vi "ABB Load-Save results.vi"(9 "confirm save":bool, 10 "Path":path, 11 "Mode":enum16{"LOAD", "Save"}(ring)) -> ()   [LabVIEW 2017]
uses:
  ABB global.vi
panel:
  in  "Case Constant\n(See Context Help)":bool=TRUE
  out "Categories":string[](array[string])
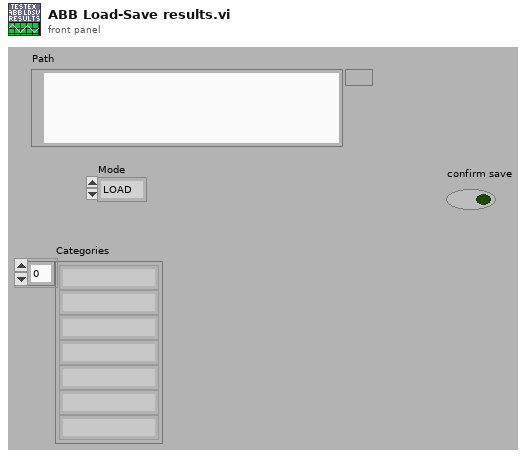
[diagram p1: front panel]
types:
  T1 = cluster{"Stator R":dbl, "Stator dT":dbl, "Rotor R":dbl, "Rotor dT":dbl, "Stator Cooling curve":dbl[][], "Rotor Cooling curve":dbl[][], "Select Resistance":enum16{"Fitted zero Res.", "Selected Res.", "Entered Res."}}
  T2 = cluster{"Stator R":dbl, "Stator dT":dbl, "Rotor R":dbl, "Rotor dT":dbl, "Stator Cooling curve":dbl[][], "Rotor Cooling curve":dbl[][], "Select Resistance":enum16{"Fitted zero Res.", "Selected Res.", "Entered Res."}}[]
  T3 = cluster{"[0]":dbl, "[1]":dbl, "[2]":dbl, "[3]":dbl, "[4]":dbl, "[5]":dbl, "[6]":dbl, "[7]":dbl}
  T4 = cluster{"DBL Array out[0]":dbl, "DBL Array out[1]":dbl, "DBL Array out[2]":dbl}
  T5 = cluster{"VT Primary":dbl, "VT Secondary":dbl, "CT  Primary":dbl, "CT Secondary":dbl, "Current Shunt":enum16{"Internal", "External"}, "Averaging interval":dbl}
  T6 = cluster{"VT Primary":dbl, "VT Secondary":dbl, "CT  Primary":dbl, "CT Secondary":dbl, "Current Shunt":enum16{"Internal", "External"}, "Avg interval":dbl}
  T7 = cluster{"temp. alloc":i32[], "category":i32[], "Category names":string[], "Category none names":string[]}
  T8 = cluster{"Number of Loads":i32, "Loads (%Rated)":dbl[]}
  T9 = enum16{"Fitted zero Res.", "Selected Res.", "Entered Res."}
  T10 = cluster{"Prior to test":dbl, "Prior v":dbl, "Prior temp":dbl, "After test":dbl, "after v":dbl, "After temp":dbl, "Test Voltage (kV)":dbl, "Test Time (min)":dbl}
  T11 = cluster{"Noise Before":string, "Noise During":string}
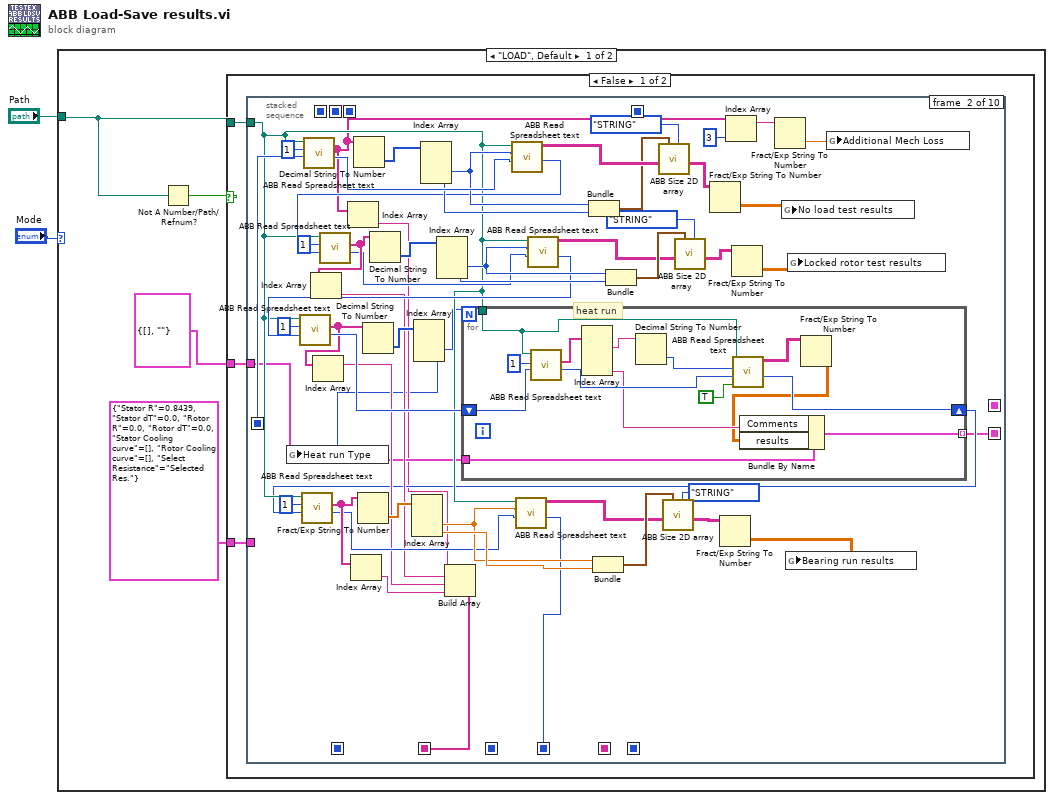
[diagram p0: block diagram]
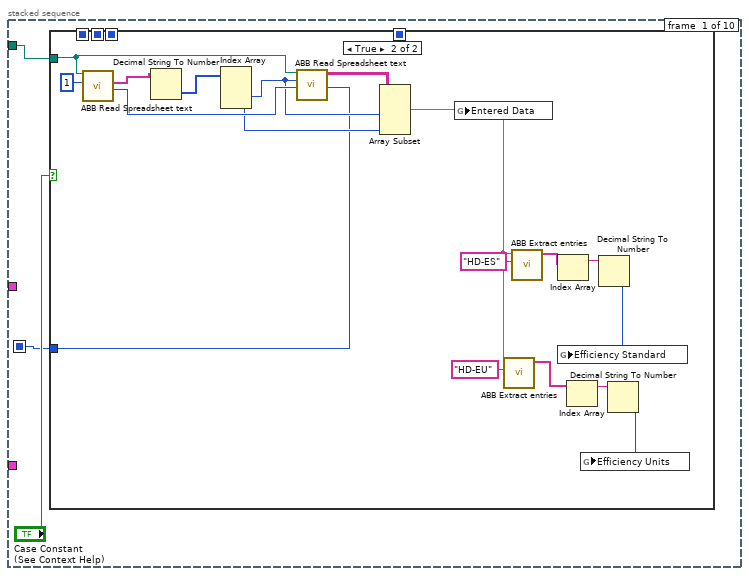
[diagram p2: hidden frame]
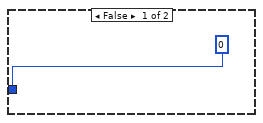
[diagram p3: hidden frame]
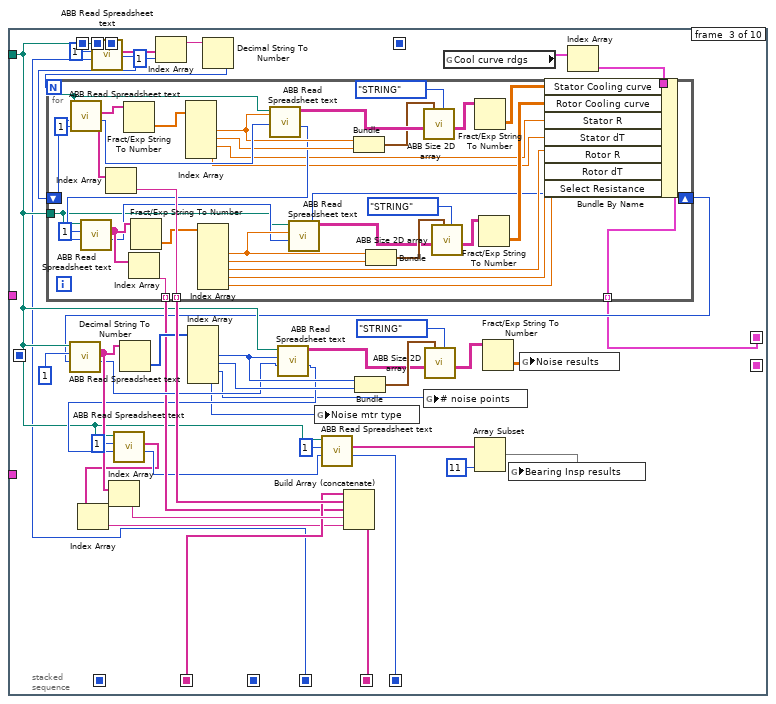
[diagram p4: hidden frame]
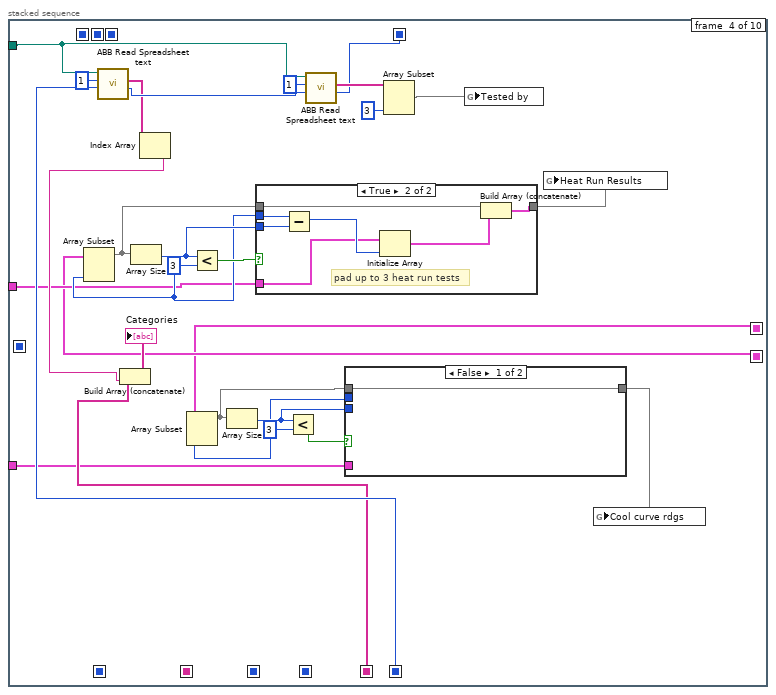
[diagram p5: hidden frame]
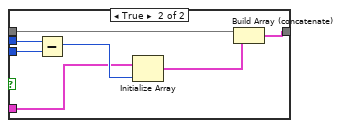
[diagram p6: hidden frame]
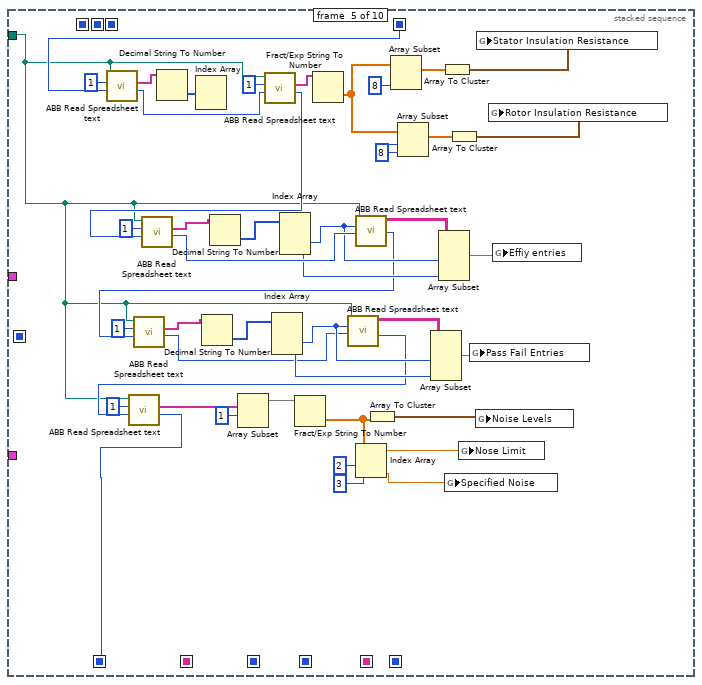
[diagram p8: hidden frame]
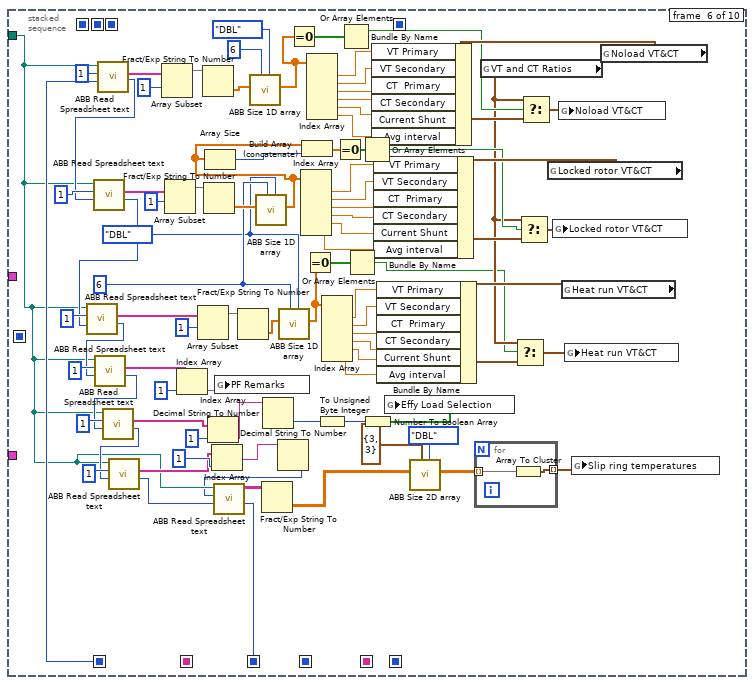
[diagram p9: hidden frame]
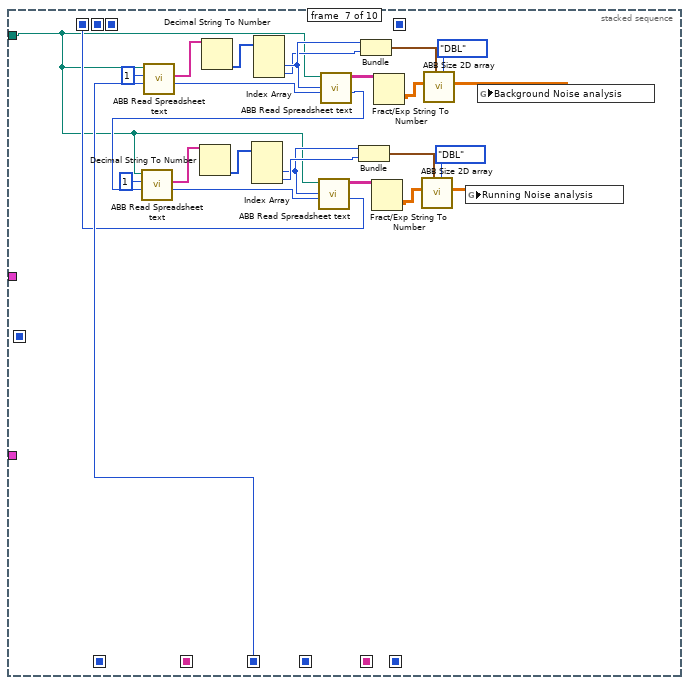
[diagram p10: hidden frame]
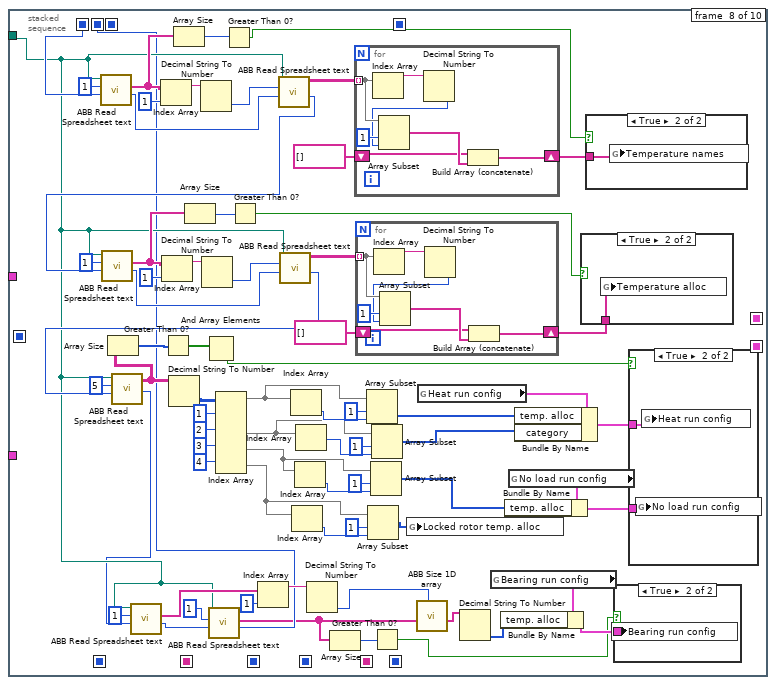
[diagram p11: hidden frame]
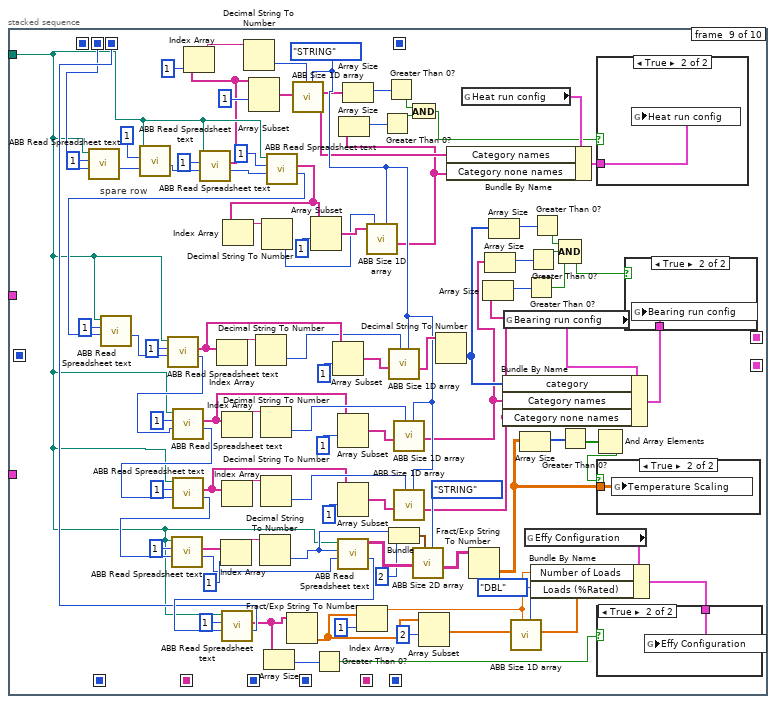
[diagram p16: hidden frame]
diagram:
  n1 = case shown="\"LOAD\", Default" "Mode" {
    tunnel: "Path" -> [w5 w638]
    frame "LOAD", Default {
      n2 = Not A Number/Path/Refnum?(number/path/refnum=w5) -> (NaN/Path/Refnum?=w6:bool)
      n3 = case shown="False" w6 {
        tunnel: w5 -> [w9 _]
        tunnel: cluster{"results":dbl[][], "Comments":string} {"results"=[], "Comments"=""} ("Heat Run") -> [w8 _]
        tunnel: T1 {"Stator R"=0.8439, "Stator dT"=0.0, "Rotor R"=0.0, "Rotor dT"=0.0, "Stator Cooling curve"=[], "Rotor Cooling curve"=[], "Select Resistance"=enum."Selected Res."} ("Cool Curve Rdgs") -> [w7 _]
        frame False {
          n4 = stacked-sequence {
            seq-local: [_ w45 _ _ _ _ _ _ _ _] -> [_ _ w111 _ _ _ _ _ _ _]
            seq-local: [_ w42 _ _ _ _ _ _ _ _] -> [_ _ w126 _ _ _ _ _ _ _]
            seq-local: [w10 _ _ _ _ _ _ _ _ _] -> [_ w75 _ _ _ _ _ _ _ _]
            seq-local: [_ _ w116 _ _ _ _ _ _ _] -> [_ _ _ w200 _ _ _ _ _ _]
            seq-local: [_ _ w114 _ _ _ _ _ _ _] -> [_ _ _ w198 _ _ _ _ _ _]
            seq-local: [_ w38 _ _ _ _ _ _ _ _] -> [_ _ _ w183 _ _ _ _ _ _]
            seq-local: [_ _ _ w182 _ _ _ _ _ _] -> [_ _ _ _ w259 _ _ _ _ _]
            seq-local: [_ _ w102 _ _ _ _ _ _ _] -> [_ _ _ w179 _ _ _ _ _ _]
            seq-local: [_ _ _ _ w223 _ _ _ _ _] -> [_ _ _ _ _ w341 _ _ _ _]
            seq-local: [_ _ _ _ _ w263 _ _ _ _] -> [_ _ _ _ _ _ w378 _ _ _]
            seq-local: [_ _ _ _ _ _ w355 _ _ _] -> [_ _ _ _ _ _ _ w407 _ _]
            seq-local: [_ _ _ _ _ _ _ w384 _ _] -> [_ _ _ _ _ _ _ _ w477 _]
            seq-local: [_ _ _ _ _ _ _ _ w503 _] -> [_ _ _ _ _ _ _ _ _ w591]
            tunnel: w9 -> [w12 w41 w112 w199 w224 w272 w354 w386 w476 w580]
            tunnel: w8 -> [_ w39 _ w184 _ _ _ _ _ _]
            tunnel: w7 -> [_ _ _ w181 _ _ _ _ _ _]
            frame #0 {
              n5 = case shown="True" "Case Constant\n(See Context Help)" {
                tunnel: [0 ("mark after read (chars.)") w23] -> w10
                tunnel: w12 -> [_ w29]
                frame False {
                }
                frame True {
                  n6 = call "ABB Read Spreadsheet text.vi"("number of rows (all:-1)"=1, "file path (dialog if empty)"=w29) -> ("mark after read (chars.)"=w30:i32, "first row"=w28:string[])  [unwired: 5 in, 3 out]
                  n7 = Decimal String To Number(string=w28) -> (number=w27:i32[])  [unwired: 2 in, 1 out]
                  n8 = Index Array(array=w27) -> (element #2=w24:i32, element #3=w25:i32)  [unwired: 3 in, 1 out]
                  n9 = call "ABB Read Spreadsheet text.vi"("start of read offset (chars.:0 )"=w30, "number of rows (all:-1)"=w24, "file path (dialog if empty)"=w29) -> ("mark after read (chars.)"=w23:i32, "all rows"=w26:string[][])  [unwired: 4 in, 3 out]
                  n10 = Array Subset(array=w26, length (row)=w24, length (col)=w25) -> (w17:string[][])  [unwired: 2 in]
                  n11 = global write "ABB global.vi" "Entered Data"(w17) -> ()
                  n12 = call "ABB Extract entries.vi"("Entry ID"="HD-EU", "Entry table in"=w17) -> ("Selected Entries"=w15:string[])  [unwired: 9 in]
                  n13 = call "ABB Extract entries.vi"("Entry ID"="HD-ES", "Entry table in"=w17) -> ("Selected Entries"=w21:string[])  [unwired: 9 in]
                  n14 = Index Array(array=w21) -> (element=w20:string)  [unwired: 1 in]
                  n15 = Index Array(array=w15) -> (element=w16:string)  [unwired: 1 in]
                  n16 = Decimal String To Number(string=w20) -> (number=w19:i32)  [unwired: 2 in, 1 out]
                  n17 = global write "ABB global.vi" "Efficiency Standard"(w19) -> ()
                  n18 = Decimal String To Number(string=w16) -> (number=w14:i32)  [unwired: 2 in, 1 out]
                  n19 = global write "ABB global.vi" "Efficiency Units"(w14) -> ()
                }
              }
            }
            frame #1 {
              n20 = call "ABB Read Spreadsheet text.vi"("start of read offset (chars.:0 )"=w75, "number of rows (all:-1)"=1, "file path (dialog if empty)"=w41) -> ("mark after read (chars.)"=w82:i32, "first row"=w35:string[])  [unwired: 4 in, 3 out]
              n21 = Index Array(array=w35) -> (element=w37:string)  [unwired: 1 in]
              n22 = Decimal String To Number(string=w35) -> (number=w81:i32[])  [unwired: 2 in, 1 out]
              n23 = Index Array(array=w81) -> (element #2=w80:i32, element #3=w79:i32)  [unwired: 3 in, 1 out]
              n24 = call "ABB Read Spreadsheet text.vi"("start of read offset (chars.:0 )"=w82, "number of rows (all:-1)"=w80, "file path (dialog if empty)"=w41) -> ("mark after read (chars.)"=w47:i32, "all rows"=w84:string[][])  [unwired: 4 in, 3 out]
              n25 = call "ABB Read Spreadsheet text.vi"("start of read offset (chars.:0 )"=w47, "number of rows (all:-1)"=1, "file path (dialog if empty)"=w41) -> ("mark after read (chars.)"=w67:i32, "first row"=w72:string[])  [unwired: 4 in, 3 out]
              n26 = Index Array(array=w72) -> (element=w43:string)  [unwired: 1 in]
              n27 = Decimal String To Number(string=w72) -> (number=w68:i32[])  [unwired: 2 in, 1 out]
              n28 = Index Array(array=w68) -> (element #2=w69:i32, element #3=w70:i32)  [unwired: 3 in, 1 out]
              n29 = call "ABB Read Spreadsheet text.vi"("start of read offset (chars.:0 )"=w67, "number of rows (all:-1)"=w69, "file path (dialog if empty)"=w41) -> ("mark after read (chars.)"=w46:i32, "all rows"=w65:string[][])  [unwired: 4 in, 3 out]
              n30 = call "ABB Read Spreadsheet text.vi"("start of read offset (chars.:0 )"=w46, "number of rows (all:-1)"=1, "file path (dialog if empty)"=w41) -> ("mark after read (chars.)"=w62:i32, "first row"=w60:string[])  [unwired: 4 in, 3 out]
              n31 = Index Array(array=w60) -> (element=w44:string)  [unwired: 1 in]
              n32 = Decimal String To Number(string=w60) -> (number=w61:i32[])  [unwired: 2 in, 1 out]
              n33 = Index Array(array=w61) -> (element #2=w36:i32)  [unwired: 3 in, 2 out]
              n34 = global write "ABB global.vi" "Heat run Type"(w36) -> ()
              n35 = for {
                N: w36 -> [_]
                tunnel: w41 -> [w98]
                shift-right: [w90] -> w40
                shift-left: w62 -> [w99]
                tunnel: w39 -> [w97]
                tunnel: [w89] -> w38 mode=indexing
                # "heat run"
                n36 = call "ABB Read Spreadsheet text.vi"("start of read offset (chars.:0 )"=w99, "number of rows (all:-1)"=1, "file path (dialog if empty)"=w98) -> ("mark after read (chars.)"=w95:i32, "first row"=w91:string[])  [unwired: 4 in, 3 out]
                n37 = Index Array(array=w91) -> (element #1=w94:string, element #4=w92:string)  [unwired: 4 in, 2 out]
                n38 = Decimal String To Number(string=w94) -> (number=w93:i32)  [unwired: 2 in, 1 out]
                n39 = call "ABB Read Spreadsheet text.vi"("remove trailng empty strings"=TRUE, "start of read offset (chars.:0 )"=w95, "number of rows (all:-1)"=w93, "file path (dialog if empty)"=w98) -> ("mark after read (chars.)"=w90:i32, "all rows"=w88:string[][])  [unwired: 3 in, 3 out]
                n40 = Fract/Exp String To Number(string=w88) -> (number=w86:dbl[][])  [unwired: 3 in, 1 out]
                n41 = Bundle By Name(cluster=w97, "Comments"=w92, "results"=w86) -> (w89:cluster{"results":dbl[][], "Comments":string})
              }
              n42 = call "ABB Read Spreadsheet text.vi"("start of read offset (chars.:0 )"=w40, "number of rows (all:-1)"=1, "file path (dialog if empty)"=w41) -> ("mark after read (chars.)"=w51:i32, "first row"=w56:string[])  [unwired: 4 in, 3 out]
              n43 = Index Array(array=w56) -> (element=w57:string)  [unwired: 1 in]
              n44 = Fract/Exp String To Number(string=w56) -> (number=w52:dbl[])  [unwired: 3 in, 1 out]
              n45 = Index Array(array=w52) -> (element #2=w53:dbl, element #3=w54:dbl)  [unwired: 3 in, 1 out]
              n46 = Build Array(w37, w43, w44, w57) -> (w42:string[])
              n47 = call "ABB Read Spreadsheet text.vi"("start of read offset (chars.:0 )"=w51, "number of rows (all:-1)"=w53, "file path (dialog if empty)"=w41) -> ("mark after read (chars.)"=w45:i32, "all rows"=w49:string[][])  [unwired: 4 in, 3 out]
              n48 = Bundle(w80, w79) -> (w83:cluster{i32, i32})  [unwired: 1 in]
              n49 = Bundle(w53, w54) -> (w50:cluster{dbl, dbl})  [unwired: 1 in]
              n50 = Bundle(w69, w70) -> (w66:cluster{i32, i32})  [unwired: 1 in]
              n51 = call "ABB Size 2D array.vi"("Type"=enum16{"Integer", "DBL", "STRING", "BOOLEAN"}."STRING", "Size"=w83, "String Array in"=w84) -> ("String Array out"=w76:string[][])  [unwired: 5 in, 3 out]
              n52 = call "ABB Size 2D array.vi"("Type"=enum16{"Integer", "DBL", "STRING", "BOOLEAN"}."STRING", "Size"=w50, "String Array in"=w49) -> ("String Array out"=w59:string[][])  [unwired: 5 in, 3 out]
              n53 = call "ABB Size 2D array.vi"("Type"=enum16{"Integer", "DBL", "STRING", "BOOLEAN"}."STRING", "Size"=w66, "String Array in"=w65) -> ("String Array out"=w74:string[][])  [unwired: 5 in, 3 out]
              n54 = Fract/Exp String To Number(string=w76) -> (number=w77:dbl[][])  [unwired: 3 in, 1 out]
              n55 = Fract/Exp String To Number(string=w59) -> (number=w58:dbl[][])  [unwired: 3 in, 1 out]
              n56 = Index Array(array=w35, index=3) -> (element=w33:string)
              n57 = Fract/Exp String To Number(string=w74) -> (number=w73:dbl[][])  [unwired: 3 in, 1 out]
              n58 = Fract/Exp String To Number(string=w33) -> (number=w32:dbl)  [unwired: 3 in, 1 out]
              n59 = global write "ABB global.vi" "No load test results"(w77) -> ()
              n60 = global write "ABB global.vi" "Bearing run results"(w58) -> ()
              n61 = global write "ABB global.vi" "Locked rotor test results"(w73) -> ()
              n62 = global write "ABB global.vi" "Additional Mech Loss"(w32) -> ()
            }
            frame #2 {
              n63 = call "ABB Read Spreadsheet text.vi"("start of read offset (chars.:0 )"=w111, "number of rows (all:-1)"=1, "file path (dialog if empty)"=w112) -> ("mark after read (chars.)"=w110:i32, "first row"=w108:string[])  [unwired: 4 in, 3 out]
              n64 = Index Array(array=w108, index=1) -> (element=w106:string)
              n65 = Decimal String To Number(string=w106) -> (number=w105:i32)  [unwired: 2 in, 1 out]
              n66 = global read "ABB global.vi" "Cool curve rdgs"() -> (w104:T2)
              n67 = Index Array(array=w104) -> (element=w103:T1)  [unwired: 1 in]
              n68 = for {
                N: w105 -> [_]
                tunnel: [w166] -> w139 mode=indexing
                tunnel: [w152] -> w125 mode=indexing
                tunnel: w103 -> [w145]
                tunnel: [w144] -> w102 mode=indexing
                tunnel: w112 -> [w143]
                shift-right: [w141] -> w109
                shift-left: w110 -> [w142]
                n69 = call "ABB Read Spreadsheet text.vi"("start of read offset (chars.:0 )"=w142, "number of rows (all:-1)"=1, "file path (dialog if empty)"=w143) -> ("mark after read (chars.)"=w171:i32, "first row"=w164:string[])  [unwired: 4 in, 3 out]
                n70 = Index Array(array=w164) -> (element=w166:string)  [unwired: 1 in]
                n71 = Fract/Exp String To Number(string=w164) -> (number=w170:dbl[])  [unwired: 3 in, 1 out]
                n72 = Index Array(array=w170) -> (element #2=w169:dbl, element #3=w168:dbl, element #4=w149:dbl, element #5=w148:dbl)  [unwired: 5 in, 1 out]
                n73 = call "ABB Read Spreadsheet text.vi"("start of read offset (chars.:0 )"=w171, "number of rows (all:-1)"=w169, "file path (dialog if empty)"=w143) -> ("mark after read (chars.)"=w153:i32, "all rows"=w173:string[][])  [unwired: 4 in, 3 out]
                n74 = call "ABB Read Spreadsheet text.vi"("start of read offset (chars.:0 )"=w153, "number of rows (all:-1)"=1, "file path (dialog if empty)"=w143) -> ("mark after read (chars.)"=w157:i32, "first row"=w163:string[])  [unwired: 4 in, 3 out]
                n75 = Index Array(array=w163) -> (element=w152:string)  [unwired: 1 in]
                n76 = Fract/Exp String To Number(string=w163) -> (number=w158:dbl[])  [unwired: 3 in, 1 out]
                n77 = Index Array(array=w158) -> (element #2=w159:dbl, element #3=w160:dbl, element #4=w147:dbl, element #5=w146:dbl, element #6=w140:dbl)  [unwired: 6 in, 1 out]
                n78 = call "ABB Read Spreadsheet text.vi"("start of read offset (chars.:0 )"=w157, "number of rows (all:-1)"=w159, "file path (dialog if empty)"=w143) -> ("mark after read (chars.)"=w141:i32, "all rows"=w155:string[][])  [unwired: 4 in, 3 out]
                n79 = Bundle(w169, w168) -> (w172:cluster{dbl, dbl})  [unwired: 1 in]
                n80 = Bundle(w159, w160) -> (w156:cluster{dbl, dbl})  [unwired: 1 in]
                n81 = call "ABB Size 2D array.vi"("Type"=enum16{"Integer", "DBL", "STRING", "BOOLEAN"}."STRING", "Size"=w172, "String Array in"=w173) -> ("String Array out"=w165:string[][])  [unwired: 5 in, 3 out]
                n82 = call "ABB Size 2D array.vi"("Type"=enum16{"Integer", "DBL", "STRING", "BOOLEAN"}."STRING", "Size"=w156, "String Array in"=w155) -> ("String Array out"=w162:string[][])  [unwired: 5 in, 3 out]
                n83 = Fract/Exp String To Number(string=w165) -> (number=w151:dbl[][])  [unwired: 3 in, 1 out]
                n84 = Fract/Exp String To Number(string=w162) -> (number=w150:dbl[][])  [unwired: 3 in, 1 out]
                n85 = Bundle By Name(cluster=w145, "Stator Cooling curve"=w151, "Rotor Cooling curve"=w150, "Stator R"=w149, "Stator dT"=w148, "Rotor R"=w147, "Rotor dT"=w146, "Select Resistance"=w140) -> (w144:T1)
              }
              n86 = call "ABB Read Spreadsheet text.vi"("start of read offset (chars.:0 )"=w109, "number of rows (all:-1)"=1, "file path (dialog if empty)"=w112) -> ("mark after read (chars.)"=w131:i32, "first row"=w138:string[])  [unwired: 4 in, 3 out]
              n87 = Index Array(array=w138) -> (element=w127:string)  [unwired: 1 in]
              n88 = Decimal String To Number(string=w138) -> (number=w132:i32[])  [unwired: 2 in, 1 out]
              n89 = Index Array(array=w132) -> (element #2=w133:i32, element #3=w134:i32, element #4=w100:i32, element #5=w101:i32)  [unwired: 5 in, 1 out]
              n90 = call "ABB Read Spreadsheet text.vi"("start of read offset (chars.:0 )"=w131, "number of rows (all:-1)"=w133, "file path (dialog if empty)"=w112) -> ("mark after read (chars.)"=w123:i32, "all rows"=w129:string[][])  [unwired: 4 in, 3 out]
              n91 = call "ABB Read Spreadsheet text.vi"("start of read offset (chars.:0 )"=w123, "number of rows (all:-1)"=1, "file path (dialog if empty)"=w112) -> ("mark after read (chars.)"=w122:i32, "first row"=w118:string[])  [unwired: 4 in, 3 out]
              n92 = Index Array(array=w118) -> (element=w117:string)  [unwired: 1 in]
              n93 = global write "ABB global.vi" "Noise mtr type"(w101) -> ()
              n94 = call "ABB Read Spreadsheet text.vi"("start of read offset (chars.:0 )"=w122, "number of rows (all:-1)"=1, "file path (dialog if empty)"=w112) -> ("mark after read (chars.)"=w116:i32, "first row"=w120:string[])  [unwired: 4 in, 3 out]
              n95 = Build Array (concatenate)(w126, w139, w125, w127, w117) -> (w114:string[])
              n96 = Bundle(w133, w134) -> (w130:cluster{i32, i32})  [unwired: 1 in]
              n97 = global write "ABB global.vi" "# noise points"(w100) -> ()
              n98 = call "ABB Size 2D array.vi"("Type"=enum16{"Integer", "DBL", "STRING", "BOOLEAN"}."STRING", "Size"=w130, "String Array in"=w129) -> ("String Array out"=w137:string[][])  [unwired: 5 in, 3 out]
              n99 = Array Subset(array=w120, length=11) -> (w121:string[])  [unwired: 1 in]
              n100 = Fract/Exp String To Number(string=w137) -> (number=w136:dbl[][])  [unwired: 3 in, 1 out]
              n101 = global write "ABB global.vi" "Bearing Insp results"(w121) -> ()
              n102 = global write "ABB global.vi" "Noise results"(w136) -> ()
            }
            frame #3 {
              w175 = 3 ("y")
              w185 = 3 ("y")
              n103 = Array Subset(array=w183, length=w185) -> (w188:cluster{"results":dbl[][], "Comments":string}[])  [unwired: 1 in]
              n104 = call "ABB Read Spreadsheet text.vi"("start of read offset (chars.:0 )"=w200, "number of rows (all:-1)"=1, "file path (dialog if empty)"=w199) -> ("mark after read (chars.)"=w201:i32, "first row"=w197:string[])  [unwired: 4 in, 3 out]
              n105 = Array Size(array=w188) -> (size(s)=w186:i32)
              n106 = Index Array(array=w197) -> (element=w196:string)  [unwired: 1 in]
              n107 = Build Array (concatenate)(w198, w196) -> (→"Categories":string[])
              n108 = Array Subset(array=w179, length=w175) -> (w178:T2)  [unwired: 1 in]
              n109 = Less?(x=w186, y=w185) -> (x < y?=w189:bool)
              n110 = Array Size(array=w178) -> (size(s)=w176:i32)
              n111 = case shown="True" w189 {
                tunnel: w188 -> [w210 w217]
                tunnel: [w210 w212] -> w187
                tunnel: w186 -> [_ w215]
                tunnel: w185 -> [_ w216]
                tunnel: w184 -> [_ w211]
                frame False {
                }
                frame True {
                  # "pad up to 3 heat run tests"
                  n112 = Subtract(x=w216, y=w215) -> (x-y=w214:i32)
                  n113 = Initialize Array(w211, w214) -> (w213:cluster{"results":dbl[][], "Comments":string}[])
                  n114 = Build Array (concatenate)(w217, w213) -> (w212:cluster{"results":dbl[][], "Comments":string}[])
                }
              }
              n115 = Less?(x=w176, y=w175) -> (x < y?=w177:bool)
              n116 = call "ABB Read Spreadsheet text.vi"("start of read offset (chars.:0 )"=w201, "number of rows (all:-1)"=1, "file path (dialog if empty)"=w199) -> ("mark after read (chars.)"=w182:i32, "first row"=w192:string[])  [unwired: 4 in, 3 out]
              n117 = case shown="False" w177 {
                tunnel: w178 -> [w202 w209]
                tunnel: [w202 w204] -> w180
                tunnel: w176 -> [_ w207]
                tunnel: w175 -> [_ w208]
                tunnel: w181 -> [_ w203]
                frame False {
                }
                frame True {
                  n118 = Subtract(x=w208, y=w207) -> (x-y=w206:i32)
                  n119 = Initialize Array(w203, w206) -> (w205:T2)
                  n120 = Build Array (concatenate)(w209, w205) -> (w204:T2)
                }
              }
              n121 = Array Subset(array=w192, length=3) -> (w190:string[])  [unwired: 1 in]
              n122 = global write "ABB global.vi" "Tested by"(w190) -> ()
              n123 = global write "ABB global.vi" "Heat Run Results"(w187) -> ()
              n124 = global write "ABB global.vi" "Cool curve rdgs"(w180) -> ()
            }
            frame #4 {
              w226 = 8 ("length")
              n125 = call "ABB Read Spreadsheet text.vi"("start of read offset (chars.:0 )"=w259, "number of rows (all:-1)"=1, "file path (dialog if empty)"=w224) -> ("mark after read (chars.)"=w258:i32, "first row"=w262:string[])  [unwired: 4 in, 3 out]
              n126 = Decimal String To Number(string=w262) -> (number=w261:i32[])  [unwired: 2 in, 1 out]
              n127 = Index Array(array=w261) -> ()  [unwired: 2 in, 2 out]
              n128 = call "ABB Read Spreadsheet text.vi"("start of read offset (chars.:0 )"=w258, "number of rows (all:-1)"=1, "file path (dialog if empty)"=w224) -> ("mark after read (chars.)"=w247:i32, "first row"=w256:string[])  [unwired: 4 in, 3 out]
              n129 = call "ABB Read Spreadsheet text.vi"("start of read offset (chars.:0 )"=w247, "number of rows (all:-1)"=1, "file path (dialog if empty)"=w224) -> ("mark after read (chars.)"=w254:i32, "first row"=w253:string[])  [unwired: 4 in, 3 out]
              n130 = Decimal String To Number(string=w253) -> (number=w252:i32[])  [unwired: 2 in, 1 out]
              n131 = Index Array(array=w252) -> (element #2=w249:i32, element #3=w250:i32)  [unwired: 3 in, 1 out]
              n132 = Fract/Exp String To Number(string=w256) -> (number=w227:dbl[])  [unwired: 3 in, 1 out]
              n133 = call "ABB Read Spreadsheet text.vi"("start of read offset (chars.:0 )"=w254, "number of rows (all:-1)"=w249, "file path (dialog if empty)"=w224) -> ("mark after read (chars.)"=w238:i32, "all rows"=w251:string[][])  [unwired: 4 in, 3 out]
              n134 = call "ABB Read Spreadsheet text.vi"("start of read offset (chars.:0 )"=w238, "number of rows (all:-1)"=1, "file path (dialog if empty)"=w224) -> ("mark after read (chars.)"=w240:i32, "first row"=w241:string[])  [unwired: 4 in, 3 out]
              n135 = Decimal String To Number(string=w241) -> (number=w242:i32[])  [unwired: 2 in, 1 out]
              n136 = Index Array(array=w242) -> (element #2=w245:i32, element #3=w244:i32)  [unwired: 3 in, 1 out]
              n137 = call "ABB Read Spreadsheet text.vi"("start of read offset (chars.:0 )"=w240, "number of rows (all:-1)"=w245, "file path (dialog if empty)"=w224) -> ("mark after read (chars.)"=w236:i32, "all rows"=w243:string[][])  [unwired: 4 in, 3 out]
              n138 = call "ABB Read Spreadsheet text.vi"("start of read offset (chars.:0 )"=w236, "number of rows (all:-1)"=1, "file path (dialog if empty)"=w224) -> ("mark after read (chars.)"=w223:i32, "first row"=w235:string[])  [unwired: 4 in, 3 out]
              n139 = Array Subset(array=w235, index=1) -> (w233:string[])  [unwired: 1 in]
              n140 = Fract/Exp String To Number(string=w233) -> (number=w222:dbl[])  [unwired: 3 in, 1 out]
              n141 = Index Array(array=w222, index #1=2 ("index"), index #2=3 ("index")) -> (element #1=w220:dbl, element #2=w219:dbl)
              n142 = Array To Cluster(array=w222) -> (cluster=w232:cluster{"[0]":dbl, "[1]":dbl})
              n143 = Array Subset(array=w227, length=8) -> (w230:dbl[])  [unwired: 1 in]
              n144 = Array Subset(array=w227, index=w226, length=w226) -> (w228:dbl[])
              n145 = Array Subset(array=w243, length (row)=w245, length (col)=w244) -> (w246:string[][])  [unwired: 2 in]
              n146 = Array Subset(array=w251, length (row)=w249, length (col)=w250) -> (w248:string[][])  [unwired: 2 in]
              n147 = Array To Cluster(array=w230) -> (cluster=w229:T3)
              n148 = global write "ABB global.vi" "Specified Noise"(w219) -> ()
              n149 = Array To Cluster(array=w228) -> (cluster=w225:T3)
              n150 = global write "ABB global.vi" "Nose Limit"(w220) -> ()
              n151 = global write "ABB global.vi" "Pass Fail Entries"(w246) -> ()
              n152 = global write "ABB global.vi" "Noise Levels"(w232) -> ()
              n153 = global write "ABB global.vi" "Stator Insulation Resistance"(w229) -> ()
              n154 = global write "ABB global.vi" "Rotor Insulation Resistance"(w225) -> ()
              n155 = global write "ABB global.vi" "Effiy entries"(w248) -> ()
            }
            frame #5 {
              w296 = 6 ("Size")
              w295 = enum16{"Integer", "DBL", "STRING", "BOOLEAN"}."DBL" ("Type")
              n156 = call "ABB Read Spreadsheet text.vi"("start of read offset (chars.:0 )"=w341, "number of rows (all:-1)"=1, "file path (dialog if empty)"=w272) -> ("mark after read (chars.)"=w317:i32, "first row"=w349:string[])  [unwired: 4 in, 3 out]
              n157 = call "ABB Read Spreadsheet text.vi"("start of read offset (chars.:0 )"=w317, "number of rows (all:-1)"=1, "file path (dialog if empty)"=w272) -> ("mark after read (chars.)"=w316:i32, "first row"=w331:string[])  [unwired: 4 in, 3 out]
              n158 = call "ABB Read Spreadsheet text.vi"("start of read offset (chars.:0 )"=w316, "number of rows (all:-1)"=1, "file path (dialog if empty)"=w272) -> ("mark after read (chars.)"=w289:i32, "first row"=w326:string[])  [unwired: 4 in, 3 out]
              n159 = call "ABB Read Spreadsheet text.vi"("start of read offset (chars.:0 )"=w289, "number of rows (all:-1)"=1, "file path (dialog if empty)"=w272) -> ("mark after read (chars.)"=w284:i32, "first row"=w288:string[])  [unwired: 4 in, 3 out]
              n160 = call "ABB Read Spreadsheet text.vi"("start of read offset (chars.:0 )"=w284, "number of rows (all:-1)"=1, "file path (dialog if empty)"=w272) -> ("mark after read (chars.)"=w275:i32, "first row"=w282:string[])  [unwired: 4 in, 3 out]
              n161 = call "ABB Read Spreadsheet text.vi"("start of read offset (chars.:0 )"=w275, "number of rows (all:-1)"=1, "file path (dialog if empty)"=w272) -> ("mark after read (chars.)"=w270:i32, "first row"=w274:string[])  [unwired: 4 in, 3 out]
              n162 = Array Subset(array=w349, index=1) -> (w351:string[])  [unwired: 1 in]
              n163 = Array Subset(array=w331, index=1) -> (w329:string[])  [unwired: 1 in]
              n164 = Index Array(array=w288, index=1) -> (element=w286:string)
              n165 = Array Subset(array=w326, index=1) -> (w328:string[])  [unwired: 1 in]
              n166 = Fract/Exp String To Number(string=w351) -> (number=w294:dbl[])  [unwired: 3 in, 1 out]
              n167 = Fract/Exp String To Number(string=w329) -> (number=w298:dbl[])  [unwired: 3 in, 1 out]
              n168 = Index Array(array=w282, index=1) -> (element=w281:string)
              n169 = Index Array(array=w274, index=1) -> (element=w273:string)
              n170 = global write "ABB global.vi" "PF Remarks"(w286) -> ()
              n171 = Fract/Exp String To Number(string=w328) -> (number=w300:dbl[])  [unwired: 3 in, 1 out]
              n172 = call "ABB Size 1D array.vi"("Type"=enum16{"Integer", "DBL", "STRING", "BOOLEAN"}."DBL", "Size"=6, "DBL Array In"=w294) -> ("DBL Array out"=w293:dbl[])  [unwired: 5 in, 3 out]
              n173 = call "ABB Size 1D array.vi"("Type"=w295, "Size"=w296, "DBL Array In"=w298) -> ("DBL Array out"=w297:dbl[])  [unwired: 5 in, 3 out]
              n174 = Array Size(array=w297) -> (size(s)=w301:i32)
              n175 = Decimal String To Number(string=w281) -> (number=w280:i32)  [unwired: 2 in, 1 out]
              n176 = Decimal String To Number(string=w273) -> (number=w271:i32)  [unwired: 2 in, 1 out]
              n177 = call "ABB Read Spreadsheet text.vi"("start of read offset (chars.:0 )"=w270, "number of rows (all:-1)"=w271, "file path (dialog if empty)"=w272) -> ("mark after read (chars.)"=w263:i32, "all rows"=w269:string[][])  [unwired: 4 in, 3 out]
              n178 = Fract/Exp String To Number(string=w269) -> (number=w267:dbl[][])  [unwired: 3 in, 1 out]
              n179 = call "ABB Size 1D array.vi"("Type"=w295, "Size"=w296, "DBL Array In"=w300) -> ("DBL Array out"=w299:dbl[])  [unwired: 5 in, 3 out]
              n180 = Equal To 0?(x=w293) -> (x = 0?=w315:bool[])
              n181 = Index Array(array=w297) -> (element #1=w334:dbl, element #2=w335:dbl, element #3=w336:dbl, element #4=w337:dbl, element #5=w338:dbl, element #6=w339:dbl)  [unwired: 6 in]
              n182 = Build Array (concatenate)(w297, w301) -> (w302:dbl[])
              n183 = Equal To 0?(x=w299) -> (x = 0?=w304:bool[])
              n184 = Index Array(array=w293) -> (element #1=w346:dbl, element #2=w345:dbl, element #3=w344:dbl, element #4=w343:dbl, element #5=w342:dbl, element #6=w340:dbl)  [unwired: 6 in]
              n185 = To Unsigned Byte Integer(number=w280) -> (unsigned 8bit integer=w278:u8)
              n186 = Index Array(array=w299) -> (element #1=w323:dbl, element #2=w322:dbl, element #3=w321:dbl, element #4=w320:dbl, element #5=w319:dbl, element #6=w318:dbl)  [unwired: 6 in]
              n187 = Equal To 0?(x=w302) -> (x = 0?=w309:bool[])
              n188 = Or Array Elements(Boolean array=w315) -> (logical OR=w313:bool)
              n189 = Or Array Elements(Boolean array=w304) -> (logical OR=w303:bool)
              n190 = Or Array Elements(Boolean array=w309) -> (logical OR=w308:bool)
              n191 = Number To Boolean Array(number=w278) -> (Boolean array=w279:bool[])
              n192 = global write "ABB global.vi" "Effy Load Selection"(w279) -> ()
              n193 = call "ABB Size 2D array.vi"("Type"=enum16{"Integer", "DBL", "STRING", "BOOLEAN"}."DBL", "Size"=cluster{"# rows":i32, "# cols":i32} {"# rows"=3, "# cols"=3}, "DBL Array In"=w267) -> ("DBL Array out"=w266:dbl[][])  [unwired: 5 in, 3 out]
              n194 = for {
                tunnel: [w353] -> w268 mode=indexing
                tunnel: w266 -> [w352] mode=indexing
                n195 = Array To Cluster(array=w352) -> (cluster=w353:T4)
              }
              n196 = global read "ABB global.vi" "VT and CT Ratios"() -> (w307:T5)
              n197 = global read "ABB global.vi" "Locked rotor VT&CT"() -> (w333:T6)
              n198 = Bundle By Name(cluster=w333, "VT Primary"=w334, "VT Secondary"=w335, "CT  Primary"=w336, "CT Secondary"=w337, "Current Shunt"=w338, "Avg interval"=w339) -> (w311:T6)
              n199 = Select(t=w307, s=w308, f=w311) -> (s? t:f=w310:T6)
              n200 = global write "ABB global.vi" "Locked rotor VT&CT"(w310) -> ()
              n201 = global read "ABB global.vi" "Heat run VT&CT"() -> (w324:T6)
              n202 = Bundle By Name(cluster=w324, "VT Primary"=w323, "VT Secondary"=w322, "CT  Primary"=w321, "CT Secondary"=w320, "Current Shunt"=w319, "Avg interval"=w318) -> (w305:T6)
              n203 = Select(t=w307, s=w303, f=w305) -> (s? t:f=w306:T6)
              n204 = global write "ABB global.vi" "Heat run VT&CT"(w306) -> ()
              n205 = global write "ABB global.vi" "Slip ring temperatures"(w268) -> ()
              n206 = global read "ABB global.vi" "Noload VT&CT"() -> (w347:T6)
              n207 = Bundle By Name(cluster=w347, "VT Primary"=w346, "VT Secondary"=w345, "CT  Primary"=w344, "CT Secondary"=w343, "Current Shunt"=w342, "Avg interval"=w340) -> (w312:T6)
              n208 = Select(t=w307, s=w313, f=w312) -> (s? t:f=w314:T6)
              n209 = global write "ABB global.vi" "Noload VT&CT"(w314) -> ()
            }
            frame #6 {
              n210 = call "ABB Read Spreadsheet text.vi"("start of read offset (chars.:0 )"=w378, "number of rows (all:-1)"=1, "file path (dialog if empty)"=w354) -> ("mark after read (chars.)"=w375:i32, "first row"=w377:string[])  [unwired: 4 in, 3 out]
              n211 = Decimal String To Number(string=w377) -> (number=w376:i32[])  [unwired: 2 in, 1 out]
              n212 = Index Array(array=w376) -> (element #2=w371:i32, element #3=w370:i32)  [unwired: 3 in, 1 out]
              n213 = call "ABB Read Spreadsheet text.vi"("start of read offset (chars.:0 )"=w375, "number of rows (all:-1)"=w371, "file path (dialog if empty)"=w354) -> ("mark after read (chars.)"=w358:i32, "all rows"=w374:string[][])  [unwired: 4 in, 3 out]
              n214 = call "ABB Read Spreadsheet text.vi"("start of read offset (chars.:0 )"=w358, "number of rows (all:-1)"=1, "file path (dialog if empty)"=w354) -> ("mark after read (chars.)"=w362:i32, "first row"=w360:string[])  [unwired: 4 in, 3 out]
              n215 = Decimal String To Number(string=w360) -> (number=w361:i32[])  [unwired: 2 in, 1 out]
              n216 = Index Array(array=w361) -> (element #2=w366:i32, element #3=w367:i32)  [unwired: 3 in, 1 out]
              n217 = call "ABB Read Spreadsheet text.vi"("start of read offset (chars.:0 )"=w362, "number of rows (all:-1)"=w366, "file path (dialog if empty)"=w354) -> ("mark after read (chars.)"=w355:i32, "all rows"=w363:string[][])  [unwired: 4 in, 3 out]
              n218 = Bundle(w366, w367) -> (w368:cluster{i32, i32})  [unwired: 1 in]
              n219 = Bundle(w371, w370) -> (w369:cluster{i32, i32})  [unwired: 1 in]
              n220 = Fract/Exp String To Number(string=w363) -> (number=w364:dbl[][])  [unwired: 3 in, 1 out]
              n221 = Fract/Exp String To Number(string=w374) -> (number=w373:dbl[][])  [unwired: 3 in, 1 out]
              n222 = call "ABB Size 2D array.vi"("Type"=enum16{"Integer", "DBL", "STRING", "BOOLEAN"}."DBL", "Size"=w368, "DBL Array In"=w364) -> ("DBL Array out"=w356:dbl[][])  [unwired: 5 in, 3 out]
              n223 = call "ABB Size 2D array.vi"("Type"=enum16{"Integer", "DBL", "STRING", "BOOLEAN"}."DBL", "Size"=w369, "DBL Array In"=w373) -> ("DBL Array out"=w357:dbl[][])  [unwired: 5 in, 3 out]
              n224 = global write "ABB global.vi" "Running Noise analysis"(w356) -> ()
              n225 = global write "ABB global.vi" "Background Noise analysis"(w357) -> ()
            }
            frame #7 {
              n226 = call "ABB Read Spreadsheet text.vi"("start of read offset (chars.:0 )"=w407, "number of rows (all:-1)"=1 ("# rows"), "file path (dialog if empty)"=w386) -> ("mark after read (chars.)"=w448:i32, "first row"=w406:string[])  [unwired: 4 in, 3 out]
              n227 = Index Array(array=w406, index=1) -> (element=w449:string)
              n228 = Array Size(array=w406) -> (size(s)=w405:i32)
              n229 = Decimal String To Number(string=w449) -> (number=w447:i32)  [unwired: 2 in, 1 out]
              n230 = Greater Than 0?(x=w405) -> (x > 0?=w404:bool)
              n231 = call "ABB Read Spreadsheet text.vi"("start of read offset (chars.:0 )"=w448, "number of rows (all:-1)"=w447, "file path (dialog if empty)"=w386) -> ("mark after read (chars.)"=w436:i32, "all rows"=w446:string[][])  [unwired: 4 in, 3 out]
              n232 = call "ABB Read Spreadsheet text.vi"("start of read offset (chars.:0 )"=w436, "number of rows (all:-1)"=1 ("# rows"), "file path (dialog if empty)"=w386) -> ("mark after read (chars.)"=w440:i32, "first row"=w403:string[])  [unwired: 4 in, 3 out]
              n233 = Index Array(array=w403, index=1) -> (element=w439:string)
              n234 = Array Size(array=w403) -> (size(s)=w402:i32)
              n235 = Decimal String To Number(string=w439) -> (number=w441:i32)  [unwired: 2 in, 1 out]
              n236 = Greater Than 0?(x=w402) -> (x > 0?=w401:bool)
              n237 = call "ABB Read Spreadsheet text.vi"("start of read offset (chars.:0 )"=w440, "number of rows (all:-1)"=w441, "file path (dialog if empty)"=w386) -> ("mark after read (chars.)"=w429:i32, "all rows"=w442:string[][])  [unwired: 4 in, 3 out]
              n238 = call "ABB Read Spreadsheet text.vi"("start of read offset (chars.:0 )"=w429, "number of rows (all:-1)"=5 ("# rows"), "file path (dialog if empty)"=w386) -> ("mark after read (chars.)"=w385:i32, "all rows"=w400:string[][])  [unwired: 4 in, 3 out]
              n239 = Array Size(array=w400) -> (size(s)=w399:i32[])
              n240 = call "ABB Read Spreadsheet text.vi"("start of read offset (chars.:0 )"=w385, "number of rows (all:-1)"=1, "file path (dialog if empty)"=w386) -> ("mark after read (chars.)"=w392:i32, "first row"=w390:string[])  [unwired: 4 in, 3 out]
              n241 = Greater Than 0?(x=w399) -> (x > 0?=w398:bool[])
              n242 = Decimal String To Number(string=w400) -> (number=w433:i32[][])  [unwired: 2 in, 1 out]
              n243 = And Array Elements(Boolean array=w398) -> (logical AND=w397:bool)
              n244 = call "ABB Read Spreadsheet text.vi"("start of read offset (chars.:0 )"=w392, "number of rows (all:-1)"=1 ("# rows"), "file path (dialog if empty)"=w386) -> ("mark after read (chars.)"=w384:i32, "first row"=w382:string[])  [unwired: 4 in, 3 out]
              n245 = Index Array(array=w433, index (row) #1=1 ("index (row)"), index (row) #2=2 ("index (row)"), index (row) #3=3 ("index (row)"), index (row) #4=4 ("index (row)")) -> (element #1=w427:i32[], element #2=w415:i32[], element #3=w413:i32[], element #4=w412:i32[])  [unwired: 4 in]
              n246 = Index Array(array=w390, index=1) -> (element=w388:string)
              n247 = Index Array(array=w427) -> (element=w428:i32)  [unwired: 1 in]
              n248 = Index Array(array=w412) -> (element=w423:i32)  [unwired: 1 in]
              n249 = Index Array(array=w413) -> (element=w424:i32)  [unwired: 1 in]
              n250 = Index Array(array=w415) -> (element=w411:i32)  [unwired: 1 in]
              n251 = Decimal String To Number(string=w388) -> (number=w387:i32)  [unwired: 2 in, 1 out]
              n252 = Array Size(array=w382) -> (size(s)=w381:i32)
              n253 = for {
                tunnel: w446 -> [w470] mode=indexing
                shift-right: [w464] -> w444
                shift-left: string[] [] -> [w465]
                n254 = Index Array(array=w470) -> (element=w468:string)  [unwired: 1 in]
                n255 = Decimal String To Number(string=w468) -> (number=w467:i32)  [unwired: 2 in, 1 out]
                n256 = Array Subset(array=w470, index=1, length=w467) -> (w466:string[])
                n257 = Build Array (concatenate)(w465, w466) -> (w464:string[])
              }
              n258 = for {
                tunnel: w442 -> [w463] mode=indexing
                shift-right: [w457] -> w435
                shift-left: string[] [] -> [w458]
                n259 = Index Array(array=w463) -> (element=w461:string)  [unwired: 1 in]
                n260 = Decimal String To Number(string=w461) -> (number=w460:i32)  [unwired: 2 in, 1 out]
                n261 = Array Subset(array=w463, index=1, length=w460) -> (w459:string[])
                n262 = Build Array (concatenate)(w458, w459) -> (w457:string[])
              }
              n263 = Array Subset(array=w427, index=1, length=w428) -> (w418:i32[])
              n264 = Array Subset(array=w412, index=1, length=w423) -> (w421:i32[])
              n265 = Array Subset(array=w413, index=1, length=w424) -> (w408:i32[])
              n266 = Array Subset(array=w415, index=1, length=w411) -> (w414:i32[])
              n267 = Greater Than 0?(x=w381) -> (x > 0?=w380:bool)
              n268 = global write "ABB global.vi" "Locked rotor temp. alloc"(w421) -> ()
              n269 = call "ABB Size 1D array.vi"("Size"=w387, "String Array in"=w382) -> ("String Array out"=w396:string[])  [unwired: 6 in, 3 out]
              n270 = global read "ABB global.vi" "Heat run config"() -> (w420:T7)
              n271 = Decimal String To Number(string=w396) -> (number=w394:i32[])  [unwired: 2 in, 1 out]
              n272 = global read "ABB global.vi" "Bearing run config"() -> (w395:T7)
              n273 = Bundle By Name(cluster=w395, "temp. alloc"=w394) -> (w393:T7)
              n274 = global read "ABB global.vi" "No load run config"() -> (w409:T7)
              n275 = Bundle By Name(cluster=w409, "temp. alloc"=w408) -> (w410:T7)
              n276 = Bundle By Name(cluster=w420, "temp. alloc"=w418, "category"=w414) -> (w419:T7)
              n277 = case shown="True" w401 {
                tunnel: w435 -> [_ w455]
                frame False {
                }
                frame True {
                  n278 = global write "ABB global.vi" "Temperature alloc"(w455) -> ()
                }
              }
              n279 = case shown="True" w404 {
                tunnel: w444 -> [_ w456]
                frame False {
                }
                frame True {
                  n280 = global write "ABB global.vi" "Temperature names"(w456) -> ()
                }
              }
              n281 = case shown="True" w380 {
                tunnel: w393 -> [_ w452]
                frame False {
                }
                frame True {
                  n282 = global write "ABB global.vi" "Bearing run config"(w452) -> ()
                }
              }
              n283 = case shown="True" w397 {
                tunnel: w419 -> [_ w454]
                tunnel: w410 -> [_ w453]
                frame False {
                }
                frame True {
                  n284 = global write "ABB global.vi" "No load run config"(w453) -> ()
                  n285 = global write "ABB global.vi" "Heat run config"(w454) -> ()
                }
              }
            }
            frame #8 {
              w527 = enum16{"Integer", "DBL", "STRING", "BOOLEAN"}."STRING" ("Type")
              # "spare row"
              n286 = call "ABB Read Spreadsheet text.vi"("start of read offset (chars.:0 )"=w477, "number of rows (all:-1)"=1 ("# rows"), "file path (dialog if empty)"=w476) -> ("mark after read (chars.)"=w562:i32)  [unwired: 4 in, 4 out]
              n287 = call "ABB Read Spreadsheet text.vi"("start of read offset (chars.:0 )"=w562, "number of rows (all:-1)"=1 ("# rows"), "file path (dialog if empty)"=w476) -> ("mark after read (chars.)"=w472:i32)  [unwired: 4 in, 4 out]
              n288 = call "ABB Read Spreadsheet text.vi"("start of read offset (chars.:0 )"=w472, "number of rows (all:-1)"=1, "file path (dialog if empty)"=w476) -> ("mark after read (chars.)"=w475:i32, "first row"=w473:string[])  [unwired: 4 in, 3 out]
              n289 = Index Array(array=w473, index=1) -> (element=w561:string)
              n290 = Decimal String To Number(string=w561) -> (number=w558:i32)  [unwired: 2 in, 1 out]
              n291 = Array Subset(array=w473, index=1) -> (w559:string[])  [unwired: 1 in]
              n292 = call "ABB Read Spreadsheet text.vi"("start of read offset (chars.:0 )"=w475, "number of rows (all:-1)"=1 ("# rows"), "file path (dialog if empty)"=w476) -> ("mark after read (chars.)"=w548:i32, "first row"=w501:string[])  [unwired: 4 in, 3 out]
              n293 = call "ABB Read Spreadsheet text.vi"("start of read offset (chars.:0 )"=w548, "number of rows (all:-1)"=1 ("# rows"), "file path (dialog if empty)"=w476) -> ("mark after read (chars.)"=w551:i32)  [unwired: 4 in, 4 out]
              n294 = call "ABB Read Spreadsheet text.vi"("start of read offset (chars.:0 )"=w551, "number of rows (all:-1)"=1 ("# rows"), "file path (dialog if empty)"=w476) -> ("mark after read (chars.)"=w531:i32, "first row"=w545:string[])  [unwired: 4 in, 3 out]
              n295 = call "ABB Read Spreadsheet text.vi"("start of read offset (chars.:0 )"=w531, "number of rows (all:-1)"=1 ("# rows"), "file path (dialog if empty)"=w476) -> ("mark after read (chars.)"=w530:i32, "first row"=w529:string[])  [unwired: 4 in, 3 out]
              n296 = call "ABB Read Spreadsheet text.vi"("start of read offset (chars.:0 )"=w530, "number of rows (all:-1)"=1 ("# rows"), "file path (dialog if empty)"=w476) -> ("mark after read (chars.)"=w523:i32, "first row"=w528:string[])  [unwired: 4 in, 3 out]
              n297 = call "ABB Read Spreadsheet text.vi"("start of read offset (chars.:0 )"=w523, "number of rows (all:-1)"=1 ("# rows"), "file path (dialog if empty)"=w476) -> ("mark after read (chars.)"=w521:i32, "first row"=w526:string[])  [unwired: 4 in, 3 out]
              n298 = Index Array(array=w545) -> (element=w543:string)  [unwired: 1 in]
              n299 = Index Array(array=w526, index=1) -> (element=w525:string)
              n300 = Index Array(array=w529) -> (element=w541:string)  [unwired: 1 in]
              n301 = Index Array(array=w528) -> (element=w532:string)  [unwired: 1 in]
              n302 = Index Array(array=w501) -> (element=w555:string)  [unwired: 1 in]
              n303 = Decimal String To Number(string=w543) -> (number=w544:i32)  [unwired: 2 in, 1 out]
              n304 = Decimal String To Number(string=w525) -> (number=w518:i32)  [unwired: 2 in, 1 out]
              n305 = Decimal String To Number(string=w541) -> (number=w540:i32)  [unwired: 2 in, 1 out]
              n306 = Decimal String To Number(string=w532) -> (number=w533:i32)  [unwired: 2 in, 1 out]
              n307 = Decimal String To Number(string=w555) -> (number=w554:i32)  [unwired: 2 in, 1 out]
              n308 = call "ABB Size 1D array.vi"("Type"=w527, "Size"=w558, "String Array in"=w559) -> ("String Array out"=w499:string[])  [unwired: 5 in, 3 out]
              n309 = Array Subset(array=w501, index=1) -> (w557:string[])  [unwired: 1 in]
              n310 = Array Subset(array=w545, index=1) -> (w547:string[])  [unwired: 1 in]
              n311 = Array Subset(array=w529, index=1) -> (w538:string[])  [unwired: 1 in]
              n312 = Array Subset(array=w528, index=1) -> (w535:string[])  [unwired: 1 in]
              n313 = call "ABB Read Spreadsheet text.vi"("start of read offset (chars.:0 )"=w521, "number of rows (all:-1)"=w518, "file path (dialog if empty)"=w476) -> ("mark after read (chars.)"=w513:i32, "all rows"=w520:string[][])  [unwired: 4 in, 3 out]
              n314 = call "ABB Read Spreadsheet text.vi"("start of read offset (chars.:0 )"=w513, "number of rows (all:-1)"=1 ("# rows"), "file path (dialog if empty)"=w476) -> ("mark after read (chars.)"=w503:i32, "first row"=w480:string[])  [unwired: 4 in, 3 out]
              n315 = Array Size(array=w480) -> (size(s)=w479:i32)
              n316 = Fract/Exp String To Number(string=w480) -> (number=w511:dbl[])  [unwired: 3 in, 1 out]
              n317 = Greater Than 0?(x=w479) -> (x > 0?=w478:bool)
              n318 = Array Size(array=w499) -> (size(s)=w502:i32)
              n319 = Index Array(array=w511, index=1) -> (element=w507:dbl)
              n320 = call "ABB Size 1D array.vi"("Type"=w527, "Size"=w554, "String Array in"=w557) -> ("String Array out"=w498:string[])  [unwired: 5 in, 3 out]
              n321 = Array Size(array=w498) -> (size(s)=w500:i32)
              n322 = Greater Than 0?(x=w500) -> (x > 0?=w496:bool)
              n323 = Greater Than 0?(x=w502) -> (x > 0?=w497:bool)
              n324 = call "ABB Size 1D array.vi"("Type"=w527, "Size"=w544, "String Array in"=w547) -> ("String Array out"=w542:string[])  [unwired: 5 in, 3 out]
              n325 = Bundle(w518, 2) -> (w516:cluster{i32, i32})  [unwired: 1 in]
              n326 = call "ABB Size 1D array.vi"("Type"=w527, "Size"=w540, "String Array in"=w538) -> ("String Array out"=w490:string[])  [unwired: 5 in, 3 out]
              n327 = call "ABB Size 1D array.vi"("Type"=w527, "Size"=w533, "String Array in"=w535) -> ("String Array out"=w489:string[])  [unwired: 5 in, 3 out]
              n328 = And(x=w497, y=w496) -> (x .and. y?=w495:bool)
              n329 = call "ABB Size 2D array.vi"("Type"=enum16{"Integer", "DBL", "STRING", "BOOLEAN"}."STRING", "Size"=w516, "String Array in"=w520) -> ("String Array out"=w515:string[][])  [unwired: 5 in, 3 out]
              n330 = Array Subset(array=w511, index=2) -> (w508:dbl[])  [unwired: 1 in]
              n331 = Decimal String To Number(string=w542) -> (number=w491:i32[])  [unwired: 2 in, 1 out]
              n332 = global read "ABB global.vi" "Heat run config"() -> (w567:T7)
              n333 = Bundle By Name(cluster=w567, "Category names"=w499, "Category none names"=w498) -> (w566:T7)
              n334 = Fract/Exp String To Number(string=w515) -> (number=w484:dbl[][])  [unwired: 3 in, 1 out]
              n335 = Array Size(array=w489) -> (size(s)=w488:i32)
              n336 = Array Size(array=w490) -> (size(s)=w487:i32)
              n337 = Array Size(array=w491) -> (size(s)=w492:i32)
              n338 = global read "ABB global.vi" "Bearing run config"() -> (w553:T7)
              n339 = Bundle By Name(cluster=w553, "category"=w491, "Category names"=w490, "Category none names"=w489) -> (w552:T7)
              n340 = call "ABB Size 1D array.vi"("Type"=enum16{"Integer", "DBL", "STRING", "BOOLEAN"}."DBL", "Size"=w507, "DBL Array In"=w508) -> ("DBL Array out"=w504:dbl[])  [unwired: 5 in, 3 out]
              n341 = Array Size(array=w484) -> (size(s)=w483:i32[])
              n342 = global read "ABB global.vi" "Effy Configuration"() -> (w509:T8)
              n343 = Greater Than 0?(x=w488) -> (x > 0?=w486:bool)
              n344 = Greater Than 0?(x=w487) -> (x > 0?=w494:bool)
              n345 = Bundle By Name(cluster=w509, "Number of Loads"=w507, "Loads (%Rated)"=w504) -> (w505:T8)
              n346 = Greater Than 0?(x=w492) -> (x > 0?=w493:bool)
              n347 = Compound Arithmetic op=AND(w493, w494, w486) -> (w485:bool)
              n348 = Greater Than 0?(x=w483) -> (x > 0?=w482:bool[])
              n349 = And Array Elements(Boolean array=w482) -> (logical AND=w481:bool)
              n350 = case shown="True" w495 {
                tunnel: w566 -> [_ w571]
                frame False {
                }
                frame True {
                  n351 = global write "ABB global.vi" "Heat run config"(w571) -> ()
                }
              }
              n352 = case shown="True" w481 {
                tunnel: w484 -> [_ w569]
                frame False {
                }
                frame True {
                  n353 = global write "ABB global.vi" "Temperature Scaling"(w569) -> ()
                }
              }
              n354 = case shown="True" w478 {
                tunnel: w505 -> [_ w568]
                frame False {
                }
                frame True {
                  n355 = global write "ABB global.vi" "Effy Configuration"(w568) -> ()
                }
              }
              n356 = case shown="True" w485 {
                tunnel: w552 -> [_ w570]
                frame False {
                }
                frame True {
                  n357 = global write "ABB global.vi" "Bearing run config"(w570) -> ()
                }
              }
            }
            frame #9 {
              n358 = call "ABB Read Spreadsheet text.vi"("start of read offset (chars.:0 )"=w591, "number of rows (all:-1)"=1 ("# rows"), "file path (dialog if empty)"=w580) -> ("mark after read (chars.)"=w633:i32)  [unwired: 4 in, 4 out]
              n359 = call "ABB Read Spreadsheet text.vi"("start of read offset (chars.:0 )"=w633, "number of rows (all:-1)"=3 ("# rows"), "file path (dialog if empty)"=w580) -> ("mark after read (chars.)"=w605:i32, "all rows"=w589:string[][])  [unwired: 4 in, 3 out]
              n360 = call "ABB Read Spreadsheet text.vi"("start of read offset (chars.:0 )"=w605, "number of rows (all:-1)"=1 ("# rows"), "file path (dialog if empty)"=w580) -> ("mark after read (chars.)"=w581:i32, "first row"=w585:string[])  [unwired: 4 in, 3 out]
              n361 = call "ABB Read Spreadsheet text.vi"("start of read offset (chars.:0 )"=w581, "number of rows (all:-1)"=1 ("# rows"), "file path (dialog if empty)"=w580) -> ("first row"=w579:string[])  [unwired: 4 in, 4 out]
              n362 = Array Size(array=w585) -> (size(s)=w584:i32)
              n363 = Array Subset(array=w585, index=1) -> (w598:string[])  [unwired: 1 in]
              n364 = Fract/Exp String To Number(string=w579) -> (number=w578:dbl[])  [unwired: 3 in, 1 out]
              n365 = Array Size(array=w589) -> (size(s)=w588:i32[])
              n366 = Greater Than 0?(x=w584) -> (x > 0?=w583:bool)
              n367 = Index Array(array=w589, index (row) #1=0 ("index (row)"), index (row) #2=1 ("index (row)"), index (row) #3=2 ("index (row)")) -> (element #1=w624:string[], element #2=w612:string[], element #3=w607:string[])  [unwired: 3 in]
              n368 = Fract/Exp String To Number(string=w598) -> (number=w603:dbl[])  [unwired: 3 in, 1 out]
              n369 = Greater Than 0?(x=w588) -> (x > 0?=w587:bool[])
              n370 = Index Array(array=w578) -> (element #2=w577:dbl, element #3=w576:dbl, element #4=w575:dbl, element #5=w574:dbl)  [unwired: 5 in, 1 out]
              n371 = Index Array(array=w603) -> (element #1=w602:dbl, element #2=w601:dbl, element #3=w600:dbl, element #4=w599:dbl, element #5=w595:dbl)  [unwired: 5 in]
              n372 = Index Array(array=w624) -> (element=w632:string)  [unwired: 1 in]
              n373 = Index Array(array=w612) -> (element=w617:string)  [unwired: 1 in]
              n374 = In Range and Coerce(upper limit=60.0, x=w595, lower limit=0.3) -> (coerced(x)=w594:dbl)  [unwired: 1 out]
              n375 = And Array Elements(Boolean array=w587) -> (logical AND=w586:bool)
              n376 = Index Array(array=w607) -> (element=w616:string)  [unwired: 1 in]
              n377 = Bundle(w577, w576) -> (w573:cluster{dbl, dbl})  [unwired: 1 in]
              n378 = Bundle(w575, w574) -> (w572:cluster{dbl, dbl})  [unwired: 1 in]
              n379 = Decimal String To Number(string=w632) -> (number=w625:i32)  [unwired: 2 in, 1 out]
              n380 = Decimal String To Number(string=w617) -> (number=w620:i32)  [unwired: 2 in, 1 out]
              n381 = global read "ABB global.vi" "VT and CT Ratios"() -> (w604:T5)
              n382 = Decimal String To Number(string=w616) -> (number=w613:i32)  [unwired: 2 in, 1 out]
              n383 = Bundle By Name(cluster=w604, "VT Primary"=w602, "VT Secondary"=w601, "CT  Primary"=w600, "CT Secondary"=w599, "Current Shunt"=w595, "Averaging interval"=w594) -> (w592:T5)
              n384 = global write "ABB global.vi" "Background Average levels (dB)"(w573) -> ()
              n385 = global write "ABB global.vi" "Running Average levels (dB)"(w572) -> ()
              n386 = Array Subset(array=w624, index=1, length=w625) -> (w629:string[])
              n387 = Array Subset(array=w612, index=1, length=w620) -> (w611:string[])
              n388 = Array Subset(array=w607, index=1, length=w613) -> (w609:string[])
              n389 = Decimal String To Number(string=w629) -> (number=w628:i32[])  [unwired: 2 in, 1 out]
              n390 = call "ABB Size 1D array.vi"("Type"=enum16{"Integer", "DBL", "STRING", "BOOLEAN"}."Integer", "Size"=w625, "Integer Array In"=w628) -> ("Integer Array Out"=w627:i32[])  [unwired: 5 in, 3 out]
              n391 = call "ABB Size 1D array.vi"("Type"=enum16{"Integer", "DBL", "STRING", "BOOLEAN"}."STRING", "Size"=w620, "String Array in"=w611) -> ("String Array out"=w610:string[])  [unwired: 5 in, 3 out]
              n392 = case shown="True" w583 {
                tunnel: w592 -> [_ w636]
                frame False {
                }
                frame True {
                  n393 = global write "ABB global.vi" "VT and CT Ratios"(w636) -> ()
                  n394 = global write "ABB global.vi" "Locked rotor VT&CT"(w636) -> ()
                  n395 = global write "ABB global.vi" "Noload VT&CT"(w636) -> ()
                  n396 = global write "ABB global.vi" "Heat run VT&CT"(w636) -> ()
                }
              }
              n397 = call "ABB Size 1D array.vi"("Type"=enum16{"Integer", "DBL", "STRING", "BOOLEAN"}."STRING", "Size"=w613, "String Array in"=w609) -> ("String Array out"=w608:string[])  [unwired: 5 in, 3 out]
              n398 = global read "ABB global.vi" "No load run config"() -> (w630:T7)
              n399 = Bundle By Name(cluster=w630, "category"=w627, "Category names"=w610, "Category none names"=w608) -> (w590:T7)
              n400 = case shown="True" w586 {
                tunnel: w590 -> [_ w637]
                frame False {
                }
                frame True {
                  n401 = global write "ABB global.vi" "No load run config"(w637) -> ()
                }
              }
            }
          }
        }
        frame True {
        }
      }
    }
    frame "Save" {
      n402 = Not A Number/Path/Refnum?(number/path/refnum=w638) -> (NaN/Path/Refnum?=w639:bool)
      n403 = case shown="False" w639 {
        tunnel: w638 -> [w640 _]
        frame False {
          n404 = stacked-sequence {
            seq-local: [_ w659 _ _ _ _ _ _ _] -> [_ _ w719 _ _ _ _ _ _]
            seq-local: [_ _ w712 _ _ _ _ _ _] -> [_ _ _ w791 _ _ _ _ _]
            seq-local: [_ _ _ w760 _ _ _ _ _] -> [_ _ _ _ w839 _ _ _ _]
            seq-local: [_ _ _ _ w797 _ _ _ _] -> [_ _ _ _ _ w860 _ _ _]
            seq-local: [_ _ _ _ _ w851 _ _ _] -> [_ _ _ _ _ _ w876 _ _]
            seq-local: [_ _ _ _ _ _ w875 _ _] -> [_ _ _ _ _ _ _ w934 _]
            seq-local: [_ _ _ _ _ _ _ w932 _] -> [_ _ _ _ _ _ _ _ w1024]
            tunnel: w640 -> [w642 _ _ _ _ _ _ _ w1022]
            frame #0 {
              n405 = File/Directory Info(path=w642) -> (size=w641:i64)  [unwired: 1 in, 6 out]
              n406 = To Long Integer(number=w641) -> (32bit integer=w645:i32)
              n407 = Not Equal To 0?(x=w645) -> (x != 0?=w644:bool)
              n408 = case shown="True" w644 {
                tunnel: "confirm save" -> [_ w647]
                tunnel: w642 -> [_ w646]
                frame False {
                }
                frame True {
                  n409 = case shown="False" w647 {
                    tunnel: w646 -> [w648 _]
                    frame False {
                      n410 = Delete(path (use dialog)=w648) -> ()  [unwired: 4 in, 3 out]
                    }
                    frame True {
                    }
                  }
                }
              }
            }
            frame #1 {
              (unwired) i16 3 ("precision (6)")
              n411 = global read "ABB global.vi" "Additional Mech Loss"() -> (w651:dbl)
              n412 = global read "ABB global.vi" "Heat Run Results"() -> (w658:cluster{"results":dbl[][], "Comments":string}[])
              n413 = global read "ABB global.vi" "Locked rotor test results"() -> (w673:dbl[][])
              n414 = global read "ABB global.vi" "Entered Data"() -> (w677:string[][])
              n415 = global read "ABB global.vi" "No load test results"() -> (w687:dbl[][])
              n416 = for {
                tunnel: w658 -> [w697] mode=indexing
                shift-right: [w692] -> w654
                shift-left: string[][] [] -> [w691]
                n417 = Unbundle By Name(w697) -> ("results"=w695:dbl[][], "Comments"=w696:string)
                n418 = Array Size(array=w695) -> (size(s)=w699:i32[])
                n419 = Number To Fractional String(number=w695, precision (6)=i16 3) -> (F-format string=w690:string[][])  [unwired: 2 in]
                n420 = Number To Decimal String(number=w699) -> (decimal integer string=w698:string[])  [unwired: 1 in]
                n421 = Build Array (concatenate)(w698, "" ("element"), w696) -> (w693:string[])
                n422 = Build Array (concatenate)(w691, w693, w690) -> (w692:string[][])
              }
              n423 = Number To Fractional String(number=w651, precision (6)=i16 4) -> (F-format string=w649:string)  [unwired: 2 in]
              n424 = Array Size(array=w677) -> (size(s)=w681:i32[])
              n425 = Array Size(array=w658) -> (size(s)=w657:i32)
              n426 = Array Size(array=w673) -> (size(s)=w675:i32[])
              n427 = Array Size(array=w687) -> (size(s)=w685:i32[])
              n428 = Number To Decimal String(number=w681) -> (decimal integer string=w679:string[])  [unwired: 1 in]
              n429 = Number To Decimal String(number=w657) -> (decimal integer string=w656:string)  [unwired: 1 in]
              n430 = Number To Decimal String(number=w675) -> (decimal integer string=w666:string[])  [unwired: 1 in]
              n431 = global read "ABB global.vi" "Bearing run results"() -> (w668:dbl[][])
              n432 = Number To Decimal String(number=w685) -> (decimal integer string=w684:string[])  [unwired: 1 in]
              n433 = Build Array (concatenate)("Entered data", w679) -> (w678:string[])
              n434 = Build Array (concatenate)("Locked Rotor Test", w666) -> (w664:string[])
              n435 = Build Array (concatenate)("No Load Test", w684, w649) -> (w683:string[])
              n436 = global read "ABB global.vi" "Heat run Type"() -> (w653:enum16{"Full Load", "Partial- & No-Load"})
              n437 = Number To Fractional String(number=w687, precision (6)=i16 3) -> (F-format string=w682:string[][])  [unwired: 2 in]
              n438 = Number To Decimal String(number=w653) -> (decimal integer string=w652:string)  [unwired: 1 in]
              n439 = Build Array (concatenate)(w678, w677) -> (w676:string[][])
              n440 = Number To Fractional String(number=w673, precision (6)=i16 3) -> (F-format string=w663:string[][])  [unwired: 2 in]
              n441 = Build Array("Heat runTest", w656, w652) -> (w662:string[])
              n442 = Array Size(array=w668) -> (size(s)=w670:i32[])
              n443 = Number To Decimal String(number=w670) -> (decimal integer string=w665:string[])  [unwired: 1 in]
              n444 = Build Array (concatenate)("Bearing Run Test", w665) -> (w661:string[])
              n445 = Number To Fractional String(number=w668, precision (6)=i16 3) -> (F-format string=w660:string[][])  [unwired: 2 in]
              n446 = Build Array (concatenate)(w676, w683, w682, w664, w663, w662, w654, w661, w660) -> (w659:string[][])
            }
            frame #2 {
              n447 = global read "ABB global.vi" "Cool curve rdgs"() -> (w709:T2)
              n448 = global read "ABB global.vi" "Noise mtr type"() -> (w702:i32)
              n449 = global read "ABB global.vi" "# noise points"() -> (w703:i32)
              n450 = for {
                tunnel: w709 -> [w735] mode=indexing
                shift-right: [w728] -> w711
                shift-left: string[][] [] -> [w729]
                n451 = Unbundle By Name(w735) -> ("Stator Cooling curve"=w745:dbl[][], "Rotor Cooling curve"=w744:dbl[][], "Stator R"=w741:dbl, "Stator dT"=w740:dbl, "Rotor R"=w737:dbl, "Rotor dT"=w736:dbl, "Select Resistance"=w727:T9)
                n452 = Array Size(array=w744) -> (size(s)=w748:i32[])
                n453 = Array Size(array=w745) -> (size(s)=w751:i32[])
                n454 = Build Array (concatenate)(w751, w741, w740) -> (w742:dbl[])
                n455 = Build Array (concatenate)(w748, w737, w736, w727) -> (w738:dbl[])
                n456 = Number To Fractional String(number=w742, precision (6)=i16 4) -> (F-format string=w750:string[])  [unwired: 2 in]
                n457 = Number To Fractional String(number=w738, precision (6)=i16 4) -> (F-format string=w749:string[])  [unwired: 2 in]
                n458 = Build Array (concatenate)("Rotor cooling curve", w749) -> (w732:string[])
                n459 = Build Array (concatenate)("Stator cooling curve", w750) -> (w734:string[])
                n460 = Number To Fractional String(number=w744, precision (6)=i16 6) -> (F-format string=w731:string[][])  [unwired: 2 in]
                n461 = Number To Fractional String(number=w745, precision (6)=i16 6) -> (F-format string=w733:string[][])  [unwired: 2 in]
                n462 = Build Array (concatenate)(w734, w733, w732, w731) -> (w730:string[][])
                n463 = Build Array (concatenate)(w729, w730) -> (w728:string[][])
              }
              n464 = Array Size(array=w709) -> (size(s)=w708:i32)
              n465 = Number To Decimal String(number=w708) -> (decimal integer string=w706:string)  [unwired: 1 in]
              n466 = global read "ABB global.vi" "Bearing Insp results"() -> (w714:string[])
              n467 = Build Array(w703, w702) -> (w701:i32[])
              n468 = Number To Decimal String(number=w701) -> (decimal integer string=w700:string[])  [unwired: 1 in]
              n469 = global read "ABB global.vi" "Noise results"() -> (w724:dbl[][])
              n470 = Build Array("Cooling Curves", w706) -> (w704:string[])
              n471 = Array Size(array=w724) -> (size(s)=w726:i32[])
              n472 = Array Size(array=w714) -> (size(s)=w717:i32)
              n473 = Number To Decimal String(number=w726) -> (decimal integer string=w722:string[])  [unwired: 1 in]
              n474 = Number To Decimal String(number=w717) -> (decimal integer string=w718:string)  [unwired: 1 in]
              n475 = Build Array (concatenate)("Noise Test", w722, w700) -> (w721:string[])
              n476 = Build Array("Bearing inspection", w718) -> (w715:string[])
              n477 = Build Array(w715, w714) -> (w713:string[][])
              n478 = Number To Fractional String(number=w724, precision (6)=i16 3) -> (F-format string=w720:string[][])  [unwired: 2 in]
              n479 = Build Array (concatenate)(w704, w711) -> (w705:string[][])
              n480 = Build Array (concatenate)(w719, w705, w721, w720, w713) -> (w712:string[][])
            }
            frame #3 {
              n481 = global read "ABB global.vi" "Specified Noise"() -> (w754:dbl)
              n482 = global read "ABB global.vi" "Pass Fail Entries"() -> (w776:string[][])
              n483 = global read "ABB global.vi" "Stator Insulation Resistance"() -> (w790:T10)
              n484 = global read "ABB global.vi" "Rotor Insulation Resistance"() -> (w763:T10)
              n485 = global read "ABB global.vi" "Noise Levels"() -> (w770:cluster{"Noise Before":dbl, "Noise During":dbl})
              n486 = global read "ABB global.vi" "Effiy entries"() -> (w778:string[][])
              n487 = global read "ABB global.vi" "Nose Limit"() -> (w759:dbl)
              n488 = global read "ABB global.vi" "Tested by"() -> (w792:string[])
              n489 = Build Array(w759, w754) -> (w755:dbl[])
              n490 = Number To Fractional String(number=w770, precision (6)=i16 3) -> (F-format string=w768:T11)  [unwired: 2 in]
              n491 = Cluster To Array(cluster=w790) -> (array=w764:dbl[])
              n492 = Array Size(array=w778) -> (size(s)=w782:i32[])
              n493 = Array Size(array=w776) -> (size(s)=w772:i32[])
              n494 = Array Size(array=w792) -> (size(s)=w795:i32)
              n495 = Number To Decimal String(number=w755, width (-)=i16 2) -> (decimal integer string=w756:string[])
              n496 = Number To Decimal String(number=w782) -> (decimal integer string=w780:string[])  [unwired: 1 in]
              n497 = Number To Decimal String(number=w772) -> (decimal integer string=w774:string[])  [unwired: 1 in]
              n498 = Cluster To Array(cluster=w768) -> (array=w766:string[])
              n499 = Cluster To Array(cluster=w763) -> (array=w761:dbl[])
              n500 = Number To Decimal String(number=w795) -> (decimal integer string=w796:string)  [unwired: 1 in]
              n501 = Build Array (concatenate)(w766, w756) -> (w757:string[])
              n502 = Build Array (concatenate)("Efficiency", w780) -> (w779:string[])
              n503 = Build Array (concatenate)("Pass-Fail", w774) -> (w775:string[])
              n504 = Build Array("Tested by", w796) -> (w793:string[])
              n505 = Build Array (concatenate)(w764, w761) -> (w762:dbl[])
              n506 = Array Size(array=w762) -> (size(s)=w788:i32)
              n507 = Build Array (concatenate)("Noise Levels", w757) -> (w765:string[])
              n508 = Build Array (concatenate)(w779, w778) -> (w777:string[][])
              n509 = Build Array (concatenate)(w775, w776) -> (w771:string[][])
              n510 = Number To Decimal String(number=w788) -> (decimal integer string=w785:string)  [unwired: 1 in]
              n511 = Number To Fractional String(number=w762, precision (6)=i16 3) -> (F-format string=w787:string[])  [unwired: 2 in]
              n512 = Build Array("HV measurements", w785) -> (w784:string[])
              n513 = Build Array(w784, w787) -> (w783:string[][])
              n514 = Build Array (concatenate)(w791, w793, w792, w783, w777, w771, w765) -> (w760:string[][])
            }
            frame #4 {
              n515 = global read "ABB global.vi" "Slip ring temperatures"() -> (w804:cluster{"K":dbl, "L":dbl, "M ":dbl}[])
              n516 = global read "ABB global.vi" "Effy Load Selection"() -> (w811:bool[])
              n517 = global read "ABB global.vi" "Locked rotor VT&CT"() -> (w828:T6)
              n518 = global read "ABB global.vi" "Heat run VT&CT"() -> (w826:T6)
              n519 = global read "ABB global.vi" "PF Remarks"() -> (w813:string)
              n520 = global read "ABB global.vi" "Noload VT&CT"() -> (w848:T6)
              n521 = Unbundle By Name(w826) -> ("VT Primary"=w825:dbl, "VT Secondary"=w824:dbl, "CT  Primary"=w823:dbl, "CT Secondary"=w822:dbl, "Current Shunt"=w819:enum16{"Internal", "External"}, "Avg interval"=w817:dbl)
              n522 = Unbundle By Name(w848) -> ("VT Primary"=w847:dbl, "VT Secondary"=w846:dbl, "CT  Primary"=w845:dbl, "CT Secondary"=w844:dbl, "Current Shunt"=w840:enum16{"Internal", "External"}, "Avg interval"=w837:dbl)
              n523 = Array Size(array=w804) -> (size(s)=w803:i32)
              n524 = Unbundle By Name(w828) -> ("VT Primary"=w829:dbl, "VT Secondary"=w830:dbl, "CT  Primary"=w831:dbl, "CT Secondary"=w832:dbl, "Current Shunt"=w836:enum16{"Internal", "External"}, "Avg interval"=w818:dbl)
              n525 = Boolean Array To Number(Boolean array=w811) -> (number=w810:u32)
              n526 = for {
                tunnel: w804 -> [w850] mode=indexing
                tunnel: [w849] -> w802 mode=indexing
                n527 = Cluster To Array(cluster=w850) -> (array=w849:dbl[])
              }
              n528 = Number To Decimal String(number=w810) -> (decimal integer string=w808:string)  [unwired: 1 in]
              n529 = Number To Decimal String(number=w803) -> (decimal integer string=w800:string)  [unwired: 1 in]
              n530 = Number To Fractional String(number=w802, precision (6)=i16 2) -> (F-format string=w798:string[][])  [unwired: 2 in]
              n531 = Build Array(w825, w824, w823, w822, w819, w817) -> (w821:dbl[])
              n532 = Build Array(w847, w846, w845, w844, w840, w837) -> (w843:dbl[])
              n533 = Build Array(w829, w830, w831, w832, w836, w818) -> (w833:dbl[])
              n534 = Number To Fractional String(number=w821) -> (F-format string=w820:string[])  [unwired: 3 in]
              n535 = Number To Fractional String(number=w843) -> (F-format string=w841:string[])  [unwired: 3 in]
              n536 = Number To Fractional String(number=w833) -> (F-format string=w835:string[])  [unwired: 3 in]
              n537 = Build Array("PF Remarks", w813) -> (w812:string[])
              n538 = Build Array("Effy load sel", w808) -> (w807:string[])
              n539 = Build Array("slip ring temp", w800) -> (w805:string[])
              n540 = Build Array (concatenate)("Heat runVT&CT", w820) -> (w815:string[])
              n541 = Build Array (concatenate)("Noload VT&CT", w841) -> (w838:string[])
              n542 = Build Array (concatenate)("Locked rotorVT&CT", w835) -> (w827:string[])
              n543 = Build Array (concatenate)(w805, w798) -> (w799:string[][])
              n544 = Build Array (concatenate)(w839, w838, w827, w815, w812, w807, w799) -> (w797:string[][])
            }
            frame #5 {
              n545 = global read "ABB global.vi" "Background Noise analysis"() -> (w866:dbl[][])
              n546 = global read "ABB global.vi" "Running Noise analysis"() -> (w854:dbl[][])
              n547 = Number To Fractional String(number=w854, precision (6)=i16 3) -> (F-format string=w852:string[][])  [unwired: 2 in]
              n548 = Number To Fractional String(number=w866, precision (6)=i16 3) -> (F-format string=w859:string[][])  [unwired: 2 in]
              n549 = Array Size(array=w852) -> (size(s)=w857:i32[])
              n550 = Array Size(array=w859) -> (size(s)=w863:i32[])
              n551 = Number To Decimal String(number=w857) -> (decimal integer string=w858:string[])  [unwired: 1 in]
              n552 = Number To Decimal String(number=w863) -> (decimal integer string=w862:string[])  [unwired: 1 in]
              n553 = Build Array (concatenate)("Running octave analysis", w858) -> (w853:string[])
              n554 = Build Array (concatenate)("Background octave analysis", w862) -> (w861:string[])
              n555 = Build Array (concatenate)(w860, w861, w859, w853, w852) -> (w851:string[][])
            }
            frame #6 {
              n556 = global read "ABB global.vi" "Locked rotor temp. alloc"() -> (w888:i32[])
              n557 = global read "ABB global.vi" "Heat run config"() -> (w884:T7)
              n558 = global read "ABB global.vi" "No load run config"() -> (w878:T7)
              n559 = global read "ABB global.vi" "Temperature names"() -> (w911:string[])
              n560 = global read "ABB global.vi" "Bearing run config"() -> (w869:T7)
              n561 = Unbundle By Name(w878) -> ("temp. alloc"=w877:i32[])
              n562 = Unbundle By Name(w884) -> ("temp. alloc"=w883:i32[], "category"=w880:i32[])
              n563 = global read "ABB global.vi" "Temperature alloc"() -> (w899:string[])
              n564 = Unbundle By Name(w869) -> ("temp. alloc"=w868:i32[])
              n565 = while {
                shift-right: [w925] -> _
                shift-left: w911 -> [w931]
                tunnel: [w926] -> w906 mode=indexing
                stop <- w923 stop-if-true
                n566 = Delete From Array(array=w931, length=8, index=0) -> (deleted portion=w927:string[], array with subset deleted=w925:string[])
                n567 = Array Size(array=w927) -> (size(s)=w929:i32)
                n568 = Number To Decimal String(number=w929) -> (decimal integer string=w928:string)  [unwired: 1 in]
                n569 = Array Size(array=w925) -> (size(s)=w924:i32)
                n570 = Build Array (concatenate)(w928, w927) -> (w926:string[])
                n571 = Equal To 0?(x=w924) -> (x = 0?=w923:bool)
              }
              n572 = while {
                shift-right: [w915] -> _
                shift-left: w899 -> [w921]
                tunnel: [w916] -> w904 mode=indexing
                stop <- w913 stop-if-true
                n573 = Delete From Array(array=w921, length=8, index=0) -> (deleted portion=w917:string[], array with subset deleted=w915:string[])
                n574 = Array Size(array=w917) -> (size(s)=w919:i32)
                n575 = Number To Decimal String(number=w919) -> (decimal integer string=w918:string)  [unwired: 1 in]
                n576 = Array Size(array=w915) -> (size(s)=w914:i32)
                n577 = Build Array (concatenate)(w918, w917) -> (w916:string[])
                n578 = Equal To 0?(x=w914) -> (x = 0?=w913:bool)
              }
              n579 = Array Size(array=w888) -> (size(s)=w889:i32)
              n580 = Array Size(array=w877) -> (size(s)=w892:i32)
              n581 = Array Size(array=w883) -> (size(s)=w893:i32)
              n582 = Array Size(array=w880) -> (size(s)=w882:i32)
              n583 = Array Size(array=w868) -> (size(s)=w871:i32)
              n584 = Build Array (concatenate)(w889, w888) -> (w890:i32[])
              n585 = Build Array (concatenate)(w892, w877) -> (w891:i32[])
              n586 = Build Array (concatenate)(w893, w883) -> (w894:i32[])
              n587 = Build Array (concatenate)(w882, w880) -> (w881:i32[])
              n588 = Number To Decimal String(number=w871) -> (decimal integer string=w873:string)  [unwired: 1 in]
              n589 = Number To Decimal String(number=w890) -> (decimal integer string=w886:string[])  [unwired: 1 in]
              n590 = Number To Decimal String(number=w891) -> (decimal integer string=w887:string[])  [unwired: 1 in]
              n591 = Build Array("Test Temp allocs") -> (w896:string[])
              n592 = Number To Decimal String(number=w894) -> (decimal integer string=w895:string[])  [unwired: 1 in]
              n593 = Number To Decimal String(number=w881) -> (decimal integer string=w879:string[])  [unwired: 1 in]
              n594 = Build Array("Bearing temp alloc", w873) -> (w872:string[])
              n595 = Number To Decimal String(number=w868) -> (decimal integer string=w870:string[])  [unwired: 1 in]
              n596 = Build Array(w872, w870) -> (w867:string[][])
              n597 = Build Array(w896, w895, w879, w887, w886) -> (w885:string[][])
              n598 = Array Size(array=w906) -> (size(s)=w910:i32[])
              n599 = Array Size(array=w904) -> (size(s)=w900:i32[])
              n600 = Number To Decimal String(number=w910) -> (decimal integer string=w908:string[])  [unwired: 1 in]
              n601 = Number To Decimal String(number=w900) -> (decimal integer string=w902:string[])  [unwired: 1 in]
              n602 = Build Array (concatenate)("Temp names", w908) -> (w907:string[])
              n603 = Build Array (concatenate)(w907, w906) -> (w905:string[][])
              n604 = Build Array (concatenate)("Temp alloc", w902) -> (w903:string[])
              n605 = Build Array (concatenate)(w903, w904) -> (w898:string[][])
              n606 = Build Array (concatenate)(w876, w905, w898, w885, w867) -> (w875:string[][])
            }
            frame #7 {
              # "spare row"
              n607 = global read "ABB global.vi" "Temperature Scaling"() -> (w980:dbl[][])
              n608 = global read "ABB global.vi" "No load run config"() -> (w964:T7)
              n609 = global read "ABB global.vi" "Effy Configuration"() -> (w972:T8)
              n610 = global read "ABB global.vi" "Bearing run config"() -> (w994:T7)
              n611 = global read "ABB global.vi" "Heat run config"() -> (w1009:T7)
              n612 = Unbundle By Name(w994) -> ("category"=w995:i32[], "Category names"=w986:string[], "Category none names"=w985:string[])
              n613 = Unbundle By Name(w964) -> ("category"=w960:i32[], "Category names"=w959:string[], "Category none names"=w933:string[])
              n614 = Unbundle By Name(w972) -> ("Number of Loads"=w971:i32, "Loads (%Rated)"=w970:dbl[])
              n615 = Unbundle By Name(w1009) -> ("Category names"=w1006:string[], "Category none names"=w1003:string[])
              n616 = Number To Fractional String(number=w980, precision (6)=i16 6) -> (F-format string=w974:string[][])  [unwired: 2 in]
              n617 = Array Size(array=w995) -> (size(s)=w996:i32)
              n618 = Array Size(array=w985) -> (size(s)=w988:i32)
              n619 = Array Size(array=w986) -> (size(s)=w989:i32)
              n620 = Array Size(array=w974) -> (size(s)=w978:i32[])
              n621 = Array Size(array=w959) -> (size(s)=w953:i32)
              n622 = Number To Decimal String(number=w996) -> (decimal integer string=w992:string)  [unwired: 1 in]
              n623 = Build Array("No load categories", "3" ("element")) -> (w958:string[])
              n624 = Number To Decimal String(number=w988) -> (decimal integer string=w987:string)  [unwired: 1 in]
              n625 = Number To Decimal String(number=w989) -> (decimal integer string=w990:string)  [unwired: 1 in]
              n626 = Array Size(array=w1006) -> (size(s)=w1008:i32)
              n627 = Build Array (concatenate)(w971, w970) -> (w969:dbl[])
              n628 = Array Size(array=w1003) -> (size(s)=w1004:i32)
              n629 = Number To Decimal String(number=w978) -> (decimal integer string=w977:string[])  [unwired: 1 in]
              n630 = Build Array("Heat run Temp categories", "2" ("element")) -> (w1001:string[])
              n631 = Build Array("") -> (w947:string[])
              n632 = Array Size(array=w933) -> (size(s)=w956:i32)
              n633 = Number To Decimal String(number=w953) -> (decimal integer string=w952:string)  [unwired: 1 in]
              n634 = Array Size(array=w960) -> (size(s)=w961:i32)
              n635 = Number To Decimal String(number=w995) -> (decimal integer string=w991:string[])  [unwired: 1 in]
              n636 = Number To Decimal String(number=w1008) -> (decimal integer string=w1007:string)  [unwired: 1 in]
              n637 = Number To Decimal String(number=w1004) -> (decimal integer string=w1005:string)  [unwired: 1 in]
              n638 = Number To Decimal String(number=w956) -> (decimal integer string=w955:string)  [unwired: 1 in]
              n639 = Build Array (concatenate)(w952, w959) -> (w949:string[])
              n640 = Build Array (concatenate)(w961, w960) -> (w951:i32[])
              n641 = Build Array (concatenate)("Temperature scaling", w977) -> (w975:string[])
              n642 = Build Array("Bearing temp alloc2", "3" ("element")) -> (w984:string[])
              n643 = Number To Fractional String(number=w969, precision (6)=i16 1) -> (F-format string=w967:string[])  [unwired: 2 in]
              n644 = Build Array (concatenate)(w992, w991) -> (w983:string[])
              n645 = Build Array (concatenate)(w987, w985) -> (w981:string[])
              n646 = Build Array (concatenate)(w990, w986) -> (w982:string[])
              n647 = Build Array (concatenate)(w955, w933) -> (w950:string[])
              n648 = Build Array (concatenate)(w1005, w1003) -> (w999:string[])
              n649 = Build Array (concatenate)(w1007, w1006) -> (w1000:string[])
              n650 = Build Array (concatenate)(w975, w974) -> (w973:string[][])
              n651 = Number To Decimal String(number=w951) -> (decimal integer string=w957:string[])  [unwired: 1 in]
              n652 = Build Array (concatenate)("Efficiencies", w967) -> (w966:string[])
              n653 = Build Array(w958, w957, w949, w950) -> (w954:string[][])
              n654 = global read "ABB global.vi" "VT and CT Ratios"() -> (w946:T5)
              n655 = Unbundle By Name(w946) -> ("VT Primary"=w945:dbl, "VT Secondary"=w944:dbl, "CT  Primary"=w943:dbl, "CT Secondary"=w942:dbl, "Current Shunt"=w941:enum16{"Internal", "External"}, "Averaging interval"=w935:dbl)
              n656 = Build Array(w945, w944, w943, w942, w941, w935) -> (w940:dbl[])
              n657 = Number To Fractional String(number=w940, precision (6)=i16 2) -> (F-format string=w937:string[])  [unwired: 2 in]
              n658 = Build Array (concatenate)("VT&CT ratios", w937) -> (w938:string[])
              n659 = Build Array (concatenate)(w1001, w1000, w999, w984, w983, w982, w981, w973, w966, w954, w938) -> (w998:string[][])
              n660 = Build Array (concatenate)(w934, w947, w998) -> (w932:string[][])
            }
            frame #8 {
              n661 = global read "ABB global.vi" "Background Average levels (dB)"() -> (w1021:cluster{"Total":dbl, "Log":dbl})
              n662 = global read "ABB global.vi" "Running Average levels (dB)"() -> (w1018:cluster{"Total":dbl, "Log":dbl})
              n663 = Unbundle(w1018) -> ("Total"=w1017:dbl, "Log"=w1016:dbl)
              n664 = Unbundle(w1021) -> ("Total"=w1020:dbl, "Log"=w1019:dbl)
              n665 = Build Array(w1020, w1019, w1017, w1016) -> (w1015:dbl[])
              n666 = Number To Fractional String(number=w1015, precision (6)=i16 2) -> (F-format string=w1013:string[])  [unwired: 2 in]
              n667 = Build Array (concatenate)("Avrg Octave levels", w1013) -> (w1011:string[])
              n668 = Build Array (concatenate)(w1024, w1011) -> (w1023:string[][])
              n669 = call "ABB Write to spreadsheet.vi"("2D data"=w1023, "file path (dialog if empty)"=w1022) -> ()  [unwired: 6 in, 1 out]
            }
          }
        }
        frame True {
        }
      }
    }
  }
